vi "VCPAM_CTRL(Host)v2.vi"() -> ()   [LabVIEW 2011]
uses:
  AlazarTech/ATS-VI/5.8.3/ATS_ctl/ATS_DMA_Channel.ctl
  <vilib>/userDefined/High Color/nirio_resource_hc.ctl
  AlazarTech/ATS-VI/5.8.3/ATS_ctl/ATS_Async_Ctrl.ctl
  AlazarTech/ATS-VI/5.8.3/ATS_ctl/Device_Ctrl.ctl
  <vilib>/FPGAPlugInAG/PCI-7830R/niLvFpga_Open_PCI-7830R.vi
  <vilib>/FPGAPlugInAG/PCI-7830R/niLvFpga_Reset_PCI-7830R.vi
  <vilib>/Utility/error.llb/Error Cluster From Error Code.vi
  <vilib>/rvi/errors/niLvFpgaAdjustHostInterfaceError.vi
  <vilib>/FPGAPlugInAG/PCI-7830R/niLvFpga_Run_PCI-7830R.vi
  <vilib>/RVI Host/nirviSupport.llb/nirviErrorClusterFromErrorCode.vi
  <vilib>/Analysis/baseanly.llb/Normalize Vector.vi
  <vilib>/FPGAPlugInAG/PCI-7830R/niLvFpga_Close_PCI-7830R.vi
  <vilib>/rvi/interface/nirviOpenFPGA/nirviOpenFPGA.xnode
  FPGA Bitfiles/VoiceCoilPAMFPGA_FPGATarget_VCPAMCTRL(FPGA)_292315D5.lvbitx
  VCPAM_CTRL(FPGA).vi
  <vilib>/rvi/interface/nirviMethod/nirviMethod.xnode
  <vilib>/rvi/interface/nirviReadWriteControl/nirviReadWriteControl.xnode
  <vilib>/rvi/interface/nirviCloseFPGA/nirviCloseFPGA.xnode
  <vilib>/Analysis/NI_AALPro.lvlib
  <vilib>/Analysis/NI_AALBase.lvlib
  <vilib>/rvi/errors/niLvFpgaMergeErrorWithErrorCode.vi
  <vilib>/FPGAPlugInAG/PCI-7830R/niLvFpga_ConfigureFifo_PCI-7830R.vi
  <vilib>/FPGAPlugInAG/PCI-7830R/niLvFpga_WriteFifo_PCI-7830R.vi
  NiFpgaLv.dll
  <vilib>/FPGAPlugInAG/PCI-7830R/niLvFpga_AcknowledgeIrq_PCI-7830R.vi
  <vilib>/rvi/interface/nirviMethod/StockFPGA_InlinedMethodWaitForMultipleIRQ.vi
  <vilib>/FPGAPlugInAG/PCI-7830R/niLvFpga_WaitOnIrq_PCI-7830R.vi
panel:
  in  "AuxPreTime":u8=15
  in  "CutTail":dbl
  in  "step_delay":u32
  in  "Phase0(deg)":dbl=82.0 format="%0.2f"
  in  "TrigPW":u32
  out "Tri_pt_sent":i32=805864
  in  "Voice Coil PAM Imaging Controller":enum32{"Main", "Tune Voice Coil", "Others"}(tab)
  in  "bscan repeat":i32=1
  in  "Savemap":bool=TRUE
  in  "even step":bool
  in  "load flow":bool
  in  "Save Setting":bool
  in  "Load SO2":bool
  out "MAP":dbl[][](graph)
  in  "MAP Disp":bool=TRUE
  in  "signal type":T1(ring)
  in  "x (mm)":dbl=5.0 format="%0.2f"
  in  "B-scan Rate":dbl=160.0 min=0.1 max=1000.0 step=0.1 format="%#_4g"
  in  "B-scan #":dbl=100.0
  in  "Y Step Size":dbl=16.0
  in  "3D scan #":dbl=300.0
  in  "Ele_Ini_Dir":bool=TRUE caption="Motor"
  in  "Elevational Mode":enum32{"Continuous", "Discrete"}(radio)
  in  "Bi_Dir_Scan":bool=TRUE
  in  "Laser Rep Rate":u32=200000
  in  "Dual Laser":bool
  out "Ele_pt_sent":i32=10978
  out "B-Scan Pos":i32=-936
  in  "Y Enable":bool=TRUE
  in  "Move x":bool
  in  "Move y":bool
  in  "Left":bool
  out "x step motor pos":i32
  in  "Pt per A-line":i32=128
  out "PLL Locked":bool
  in  "Channel":T2
  in  "Trig. Delay (us)":sgl=4.3
  out "DAQ Error":bool
  out "Error source":string="ATS :     ApiSuccess"
  in  "Display Data Per             Frm":bool=TRUE
  in  "file path":path=path "C:/Users/MEMS-PAM/My Data/2013-03-07/2.dat"
  in  "Save Data":bool=TRUE
  in  "acc_PA":bool=TRUE
  out "B-scan saved":i32=684
  out "B-scan displayed":i32=684
  in  "EveryFrm":i32 format="%b"
  in  "Pulse_Out_En":bool
  out "B-Scan":u16[][](graph)
  out "Alines":i32=1176
  in  "start":i32
  in  "depth":i32=128
  out "PD":u16[](graph)
  in  "Ele_StepM_En":bool
  in  "xsteps":i32
  in  "x0 (mm)":dbl format="%0.4f"
  out "x-y":u32=36
  in  "catbscan":i16=6
  in  "stop":bool
  out "data_fetch_finished":bool
  out "stop_disp":bool=TRUE
  in  "showmap":bool=TRUE
  in  "A/B-line show":bool=TRUE
  out "Vocie-coil Traj":i16[](graph)=[6490, 6495, 6499, 6504, 6508, 6512, 6516, 6519, 6523, 6526, 6529, 6532, 6535, 6537, 6540, 6542, 6544, 6546, 6547, 6549, 6550, 6551, 6552, 6553, 6553, 6553, 6554, 6554, 6553, 6553, 6552, 6551, 6550, 6549, 6548, 6546, 6544, 6543, 6540, 6538, 6536, 6533, 6530, 6527, 6524, 6520, 6517, 6513, 6509, 6505, 6500, 6496, 6491, 6486, 6481, 6476, 6470, 6465, 6459, 6453, 6447, 6440, 6434, 6427, 6420, 6413, 6405, 6398, 6390, 6382, 6374, 6366, 6358, 6349, 6340, 6331, 6322, 6313, 6304, 6294, 6284, 6274, 6264, 6253, 6243, 6232, 6221, 6210, 6199, 6187, 6176, 6164, 6152, 6140, 6127, 6115, 6102, 6089, 6076, 6063, 6050, 6036, 6023, 6009, 5995, 5980, 5966, 5951, 5937, 5922, 5907, 5891, 5876, 5860, 5845, 5829, 5813, 5796, 5780, 5763, 5747, 5730, 5713, 5695, 5678, 5660, 5643, 5625, 5607, 5588, 5570, 5552, 5533, 5514, 5495, 5476, 5457, 5437, 5417, 5398, 5378, 5358, 5337, 5317, 5296, 5276, 5255, 5234, 5213, 5191, 5170, 5148, 5127, 5105, 5083, 5061, 5038, 5016, 4993, 4970, 4948, 4925, 4901, 4878, 4855, 4831, 4807, 4783, 4759, 4735, 4711, 4687, 4662, 4637, 4613, 4588, 4563, 4537, 4512, 4487, 4461, 4435, 4409, 4383, 4357, 4331, 4305, 4278, 4252, 4225, 4198, 4171, 4144, 4117, 4090, 4062, 4035, 4007, 3979, 3952, 3924, 3895, 3867, 3839, 3810, 3782, 3753, 3724, 3696, 3667, 3638, 3608, 3579, 3550, 3520, 3491, 3461, 3431, 3401, 3371, 3341, 3311, 3281, 3250, 3220, 3189, 3159, 3128, 3097, 3066, 3035, 3004, 2973, 2942, 2911, 2879, 2848, 2816, 2784, 2753, 2721, 2689, 2657, 2625, 2593, 2561, 2528, 2496, 2464, 2431, 2399, 2366, 2333, 2301, 2268, 2235, 2202, 2169, 2136, 2103, 2070, 2036, 2003, 1970, 1936, 1903, 1869, 1836, 1802, 1768, 1734, 1701, 1667, 1633, 1599, 1565, 1531, 1497, 1463, 1429, 1395, 1360, 1326, 1292, 1257, 1223, 1189, 1154, 1120, 1085, 1051, 1016, 981, 947, 912, 877, 843, 808, 773, 738, 704, 669, 634, 599, 564, 529, 494, 459, 425, 390, 355, 320, 285, 250, 215, 180, 145, 110, 75, 40, 5, -30, -65, -100, -135, -170, -205, -240, -275, -310, -345, -380, -415, -450, -485, -520, -555, -590, -625, -659, -694, -729, -764, -799, -833, -868, -903, -938, -972, -1007, -1041, -1076, -1110, -1145, -1179, -1214, -1248, -1283, -1317, -1351, -1385, -1420, -1454, -1488, -1522, -1556, -1590, -1624, -1658, -1692, -1725, -1759, -1793, -1827, -1860, -1894, -1927, -1961, -1994, -2027, -2061, -2094, -2127, -2160, -2193, -2226, -2259, -2292, -2325, -2357, -2390, -2423, -2455, -2487, -2520, -2552, -2584, -2616, -2649, -2681, -2712, -2744, -2776, -2808, -2839, -2871, -2902, -2934, -2965, -2996, -3027, -3058, -3089, -3120, -3151, -3181, -3212, -3242, -3273, -3303, -3333, -3363, -3393, -3423, -3453, -3483, -3512, -3542, -3571, -3601, -3630, -3659, -3688, -3717, -3746, -3774, -3803, -3831, -3860, -3888, -3916, -3944, -3972, -4000, -4027, -4055, -4082, -4110, -4137, -4164, -4191, -4218, -4245, -4271, -4298, -4324, -4350, -4377, -4403, -4428, -4454, -4480, -4505, -4531, -4556, -4581, -4606, -4631, -4656, -4680, -4705, -4729, -4753, -4777, -4801, -4825, -4848, -4872, -4895, -4918, -4941, -4964, -4987, -5010, -5032, -5055, -5077, -5099, -5121, -5143, -5164, -5186, -5207, -5228, -5249, -5270, -5291, -5312, -5332, -5352, -5372, -5392, -5412, -5432, -5451, -5471, -5490, -5509, -5528, -5547, -5565, -5584, -5602, -5620, -5638, -5656, -5673, -5691, -5708, -5725, -5742, -5759, -5775, -5792, -5808, -5824, -5840, -5856, -5872, -5887, -5903, -5918, -5933, -5947, -5962, -5977, -5991, -6005, -6019, -6033, -6046, -6060, -6073, -6086, -6099, -6112, -6124, -6137, -6149, -6161, -6173, -6184, -6196, -6207, -6218, -6229, -6240, -6251, -6261, -6271, -6281, -6291, -6301, -6311, -6320, -6329, -6338, -6347, -6356, -6364, -6372, -6380, -6388, -6396, -6404, -6411, -6418, -6425, -6432, -6438, -6445, -6451, -6457, -6463, -6469, -6474, -6480, -6485, -6490, -6495, -6499, -6504, -6508, -6512, -6516, -6519, -6523, -6526, -6529, -6532, -6535, -6537, -6540, -6542, -6544, -6546, -6547, -6549, -6550, -6551, -6552, -6553, -6553, -6553, -6554, -6554, -6553, -6553, -6552, -6551, -6550, -6549, -6548, -6546, -6544, -6543, -6540, -6538, -6536, -6533, -6530, -6527, -6524, -6520, -6517, -6513, -6509, -6505, -6500, -6496, -6491, -6486, -6481, -6476, -6470, -6465, -6459, -6453, -6447, -6440, -6434, -6427, -6420, -6413, -6405, -6398, -6390, -6382, -6374, -6366, -6358, -6349, -6340, -6331, -6322, -6313, -6304, -6294, -6284, -6274, -6264, -6253, -6243, -6232, -6221, -6210, -6199, -6187, -6176, -6164, -6152, -6140, -6127, -6115, -6102, -6089, -6076, -6063, -6050, -6036, -6023, -6009, -5995, -5980, -5966, -5951, -5937, -5922, -5907, -5891, -5876, -5860, -5845, -5829, -5813, -5796, -5780, -5763, -5747, -5730, -5713, -5695, -5678, -5660, -5643, -5625, -5607, -5588, -5570, -5552, -5533, -5514, -5495, -5476, -5457, -5437, -5417, -5398, -5378, -5358, -5337, -5317, -5296, -5276, -5255, -5234, -5213, -5191, -5170, -5148, -5127, -5105, -5083, -5061, -5038, -5016, -4993, -4970, -4948, -4925, -4901, -4878, -4855, -4831, -4807, -4783, -4759, -4735, -4711, -4687, -4662, -4637, -4613, -4588, -4563, -4537, -4512, -4487, -4461, -4435, -4409, -4383, -4357, -4331, -4305, -4278, -4252, -4225, -4198, -4171, -4144, -4117, -4090, -4062, -4035, -4007, -3979, -3952, -3924, -3895, -3867, -3839, -3810, -3782, -3753, -3724, -3696, -3667, -3638, -3608, -3579, -3550, -3520, -3491, -3461, -3431, -3401, -3371, -3341, -3311, -3281, -3250, -3220, -3189, -3159, -3128, -3097, -3066, -3035, -3004, -2973, -2942, -2911, -2879, -2848, -2816, -2784, -2753, -2721, -2689, -2657, -2625, -2593, -2561, -2528, -2496, -2464, -2431, -2399, -2366, -2333, -2301, -2268, -2235, -2202, -2169, -2136, -2103, -2070, -2036, -2003, -1970, -1936, -1903, -1869, -1836, -1802, -1768, -1734, -1701, -1667, -1633, -1599, -1565, -1531, -1497, -1463, -1429, -1395, -1360, -1326, -1292, -1257, -1223, -1189, -1154, -1120, -1085, -1051, -1016, -981, -947, -912, -877, -843, -808, -773, -738, -704, -669, -634, -599, -564, -529, -494, -459, -425, -390, -355, -320, -285, -250, -215, -180, -145, -110, -75, -40, -5, 30, 65, 100, 135, 170, 205, 240, 275, 310, 345, 380, 415, 450, 485, 520, 555, 590, 625, 659, 694, 729, 764, 799, 833, 868, 903, 938, 972, 1007, 1041, 1076, 1110, 1145, 1179, 1214, 1248, 1283, 1317, 1351, 1385, 1420, 1454, 1488, 1522, 1556, 1590, 1624, 1658, 1692, 1725, 1759, 1793, 1827, 1860, 1894, 1927, 1961, 1994, 2027, 2061, 2094, 2127, 2160, 2193, 2226, 2259, 2292, 2325, 2357, 2390, 2423, 2455, 2487, 2520, 2552, 2584, 2616, 2649, 2681, 2712, 2744, 2776, 2808, 2839, 2871, 2902, 2934, 2965, 2996, 3027, 3058, 3089, 3120, 3151, 3181, 3212, 3242, 3273, 3303, 3333, 3363, 3393, 3423, 3453, 3483, 3512, 3542, 3571, 3601, 3630, 3659, 3688, 3717, 3746, 3774, 3803, 3831, 3860, 3888, 3916, 3944, 3972, 4000, 4027, 4055, 4082, 4110, 4137, 4164, 4191, 4218, 4245, 4271, 4298, 4324, 4350, 4377, 4403, 4428, 4454, 4480, 4505, 4531, 4556, 4581, 4606, 4631, 4656, 4680, 4705, 4729, 4753, 4777, 4801, 4825, 4848, 4872, 4895, 4918, 4941, 4964, 4987, 5010, 5032, 5055, 5077, 5099, 5121, 5143, 5164, 5186, 5207, 5228, 5249, 5270, 5291, 5312, 5332, 5352, 5372, 5392, 5412, 5432, 5451, 5471, 5490, 5509, 5528, 5547, 5565, 5584, 5602, 5620, 5638, 5656, 5673, 5691, 5708, 5725, 5742, 5759, 5775, 5792, 5808, 5824, 5840, 5856, 5872, 5887, 5903, 5918, 5933, 5947, 5962, 5977, 5991, 6005, 6019, 6033, 6046, 6060, 6073, 6086, 6099, 6112, 6124, 6137, 6149, 6161, 6173, 6184, 6196, 6207, 6218, 6229, 6240, 6251, 6261, 6271, 6281, 6291, 6301, 6311, 6320, 6329, 6338, 6347, 6356, 6364, 6372, 6380, 6388, 6396, 6404, 6411, 6418, 6425, 6432, 6438, 6445, 6451, 6457, 6463, 6469, 6474, 6480, 6485]
  out "VC_POS":i16[](graph)
  in  "AcqVCPos":bool
  in  "Calc_delay":bool
  out "VC_In":dbl[](graph)=[1.0, 0.9999857270394815, 0.999942908565361, 0.9998715457999312, 0.999771640780308, 0.9996431963583721, 0.9994862162006879, 0.9993007047883986, 0.9990866674170983, 0.9988441101966808, 0.9985730400511657, 0.9982734647184995, 0.9979453927503363, 0.9975888335117926, 0.9972037971811801, 0.9967902947497157, 0.9963483380212069, 0.9958779396117159, 0.9953791129491981, 0.9948518722731206, 0.9942962326340535, 0.9937122098932426, 0.9930998207221545, 0.9924590826020026, 0.991790013823246, 0.99109263348507, 0.990366961494838, 0.9896130185675259, 0.9888308262251285, 0.988020406796047, 0.9871817834144501, 0.9863149800196149, 0.9854200213552425, 0.9844969329687524, 0.9835457412105527, 0.9825664732332882, 0.9815591569910653, 0.9805238212386539, 0.9794604955306667, 0.9783692102207152, 0.977249996460544, 0.9761028861991403, 0.9749279121818236, 0.9737251079493088, 0.9724945078367512, 0.9712361469727636, 0.9699500612784169, 0.9686362874662107, 0.9672948630390295, 0.9659258262890681, 0.9645292162967425, 0.9631050729295701, 0.9616534368410363, 0.960174349469429, 0.9586678530366607, 0.9571339905470584, 0.9555728057861408, 0.9539843433193637, 0.9523686484908522, 0.9507257674221025, 0.9490557470106686, 0.9473586349288206, 0.9456344796221867, 0.9438833303083672, 0.9421052369755334, 0.9403002503809957, 0.9384684220497604, 0.936609804273053, 0.9347244501068311, 0.9328124133702644, 0.9308737486442044, 0.9289085112696193, 0.9269167573460219, 0.9248985437298606, 0.9228539280329038, 0.9207829686205878, 0.9186857246103585, 0.9165622558699758, 0.9144126230158125, 0.9122368874111166, 0.9100351111642666, 0.9078073571269917, 0.9055536888925844, 0.9032741707940783, 0.9009688679024191, 0.8986378460245992, 0.8962811717017867, 0.8938989122074191, 0.8914911355452896, 0.8890579104475989, 0.8865993063730001, 0.8841153935046094, 0.8816062427480091, 0.8790719257292169, 0.8765125147926478, 0.8739280829990428, 0.8713187041233894, 0.8686844526528094, 0.8660254037844387, 0.8633416334232749, 0.8606332181800164, 0.8579002353688691, 0.8551427630053463, 0.8523608798040346, 0.849554665176354, 0.8467241992282839, 0.8438695627580834, 0.8409908372539782, 0.8380881048918408, 0.8351614485328384, 0.832210951721074, 0.8292366986811948, 0.826238774315995, 0.8232172642039852, 0.820172254596956, 0.8171038324175097, 0.814012085256585, 0.8108971013709507, 0.8077589696806924, 0.8045977797666681, 0.8014136218679567, 0.798206586879277, 0.7949767663483978, 0.7917242524735195, 0.7884491381006479, 0.7851515167209376, 0.7818314824680299, 0.7784891301153587, 0.7751245550734519, 0.7717378533872015, 0.7683291217331278, 0.7648984574166141, 0.7614459583691345, 0.7579717231454527, 0.7544758509208145, 0.750958441488111, 0.7474195952550354, 0.7438594132412116, 0.7402779970753156, 0.736675448992169, 0.7330518718298265, 0.7294073690266338, 0.7257420446182822, 0.7220560032348308, 0.7183493500977277, 0.714622191016799, 0.7108746323872351, 0.7071067811865472, 0.7033187449715197, 0.6995106318751337, 0.6956825506034865, 0.6918346104326822, 0.6879669212057188, 0.6840795933293458, 0.6801727377709195, 0.6762464660552285, 0.6723008902613169, 0.668336123019278, 0.6643522775070462, 0.660349467447159, 0.6563278071035183, 0.6522874112781208, 0.6482283953077885, 0.644150875060869, 0.640054966933935, 0.6359407878484549, 0.6318084552474614, 0.6276580870921933, 0.6234898018587336, 0.6193037185346221, 0.615099956615464, 0.610878636101514, 0.6066398774942554, 0.6023838017929554, 0.5981105304912161, 0.5938201855735014, 0.5895128895116599, 0.5851887652614235, 0.580847936258903, 0.5764905264170588, 0.5721166601221698, 0.5677264622302762, 0.5633200580636222, 0.5588975734070712, 0.554459134504523, 0.5500048680553021, 0.5455349012105488, 0.5410493615695817, 0.5365483771762631, 0.5320320765153362, 0.527500588508765, 0.5229540425120464, 0.5183925683105252, 0.5138162961156819, 0.5092253565614233, 0.5046198807003452, 0.5000000000000002, 0.49536584633913555, 0.49071755200393813, 0.48605524968424857, 0.4813790724697832, 0.47668915384632504, 0.47198562769192326, 0.46726862827306165, 0.46253829024083554, 0.45779474862709846, 0.4530381388406172, 0.4482685966631967, 0.4434862582458137, 0.4386912601047207, 0.4338837391175584, 0.4290638325194388, 0.4242316778990376, 0.41938741319465644, 0.41453117669029566, 0.4096631070116965, 0.40478334312239406, 0.39989202431974064, 0.39498929023093887, 0.3900752808090466, 0.38515013632899103, 0.3802139973835553, 0.37526700487937437, 0.3703093000329032, 0.36534102436639526, 0.360362319703853, 0.355373328166989, 0.3503741921711594, 0.3453650544213078, 0.34034605790788275, 0.3353173459027645, 0.33027906195516676, 0.32523134988754737, 0.3201743537914943, 0.31510821802362093, 0.3100330872014367, 0.3049491061992275, 0.29985642014391134, 0.2947551744109045, 0.2896455146199625, 0.2845275866310327, 0.27940153654008093, 0.2742675106749307, 0.26912565559107654, 0.2639761180675101, 0.25881904510252046, 0.2536545839095077, 0.2484828819127708, 0.24330408674330897, 0.23811834623459788, 0.23292580841837887, 0.22772662152042417, 0.22252093395631467, 0.2173088943271943, 0.21209065141553693, 0.20686635418089053, 0.20163615175563354, 0.19640019344070933, 0.19115862870137254, 0.18591160716291433, 0.1806592786063992, 0.17540179296438138, 0.17013930031663288, 0.16487195088585127, 0.15959989503337946, 0.15432328325490557, 0.1490422661761747, 0.14375699454868143, 0.13846761924537423, 0.13317429125634095, 0.12787716168450625, 0.12257638174131076, 0.117272102742402, 0.11196447610330765, 0.10665365333512039, 0.10133978604016586, 0.096023025907682, 0.09070352470948198, 0.08538143429562871, 0.08005690659009315, 0.07473009358642448, 0.06940114734340436, 0.06407021998071315, 0.058737463674580714, 0.053403030653449146, 0.048067073193620594, 0.042729743614917, 0.03739119427632544, 0.03205157757165539, 0.02671104592518208, 0.02136975178730176, 0.01602784763017357, 0.010685485943373305, 0.005342819229534299, 2.0499976092743302e-16, -0.005342819229534634, -0.010685485943372895, -0.016027847630173904, -0.021369751787301352, -0.026711045925182413, -0.03205157757165498, -0.03739119427632577, -0.04272974361491659, -0.04806707319362093, -0.05340303065344874, -0.05873746367458105, -0.06407021998071273, -0.06940114734340469, -0.07473009358642406, -0.08005690659009349, -0.08538143429562829, -0.09070352470948231, -0.09602302590768158, -0.10133978604016619, -0.10665365333511997, -0.11196447610330798, -0.1172721027424016, -0.1225763817413111, -0.12787716168450583, -0.13317429125634128, -0.13846761924537382, -0.14375699454868177, -0.14904226617617428, -0.1543232832549059, -0.15959989503337907, -0.1648719508858516, -0.1701393003166325, -0.17540179296438171, -0.1806592786063988, -0.18591160716291466, -0.19115862870137215, -0.19640019344070966, -0.20163615175563315, -0.20686635418089086, -0.21209065141553654, -0.21730889432719463, -0.22252093395631428, -0.2277266215204245, -0.23292580841837848, -0.2381183462345982, -0.24330408674330858, -0.24848288191277113, -0.2536545839095073, -0.2588190451025208, -0.2639761180675097, -0.2691256555910769, -0.2742675106749303, -0.27940153654008126, -0.28452758663103234, -0.28964551461996285, -0.2947551744109041, -0.2998564201439117, -0.3049491061992271, -0.310033087201437, -0.31510821802362055, -0.3201743537914946, -0.325231349887547, -0.3302790619551671, -0.33531734590276413, -0.3403460579078831, -0.34536505442130744, -0.3503741921711597, -0.35537332816698863, -0.36036231970385335, -0.3653410243663949, -0.3703093000329035, -0.375267004879374, -0.38021399738355566, -0.38515013632899064, -0.3900752808090469, -0.3949892902309385, -0.39989202431974097, -0.40478334312239367, -0.40966310701169684, -0.41453117669029527, -0.4193874131946568, -0.4242316778990372, -0.42906383251943914, -0.433883739117558, -0.43869126010472104, -0.44348625824581334, -0.448268596663197, -0.45303813884061683, -0.4577947486270988, -0.46253829024083515, -0.467268628273062, -0.47198562769192287, -0.4766891538463254, -0.4813790724697828, -0.4860552496842489, -0.49071755200393774, -0.4953658463391359, -0.49999999999999983, -0.5046198807003456, -0.509225356561423, -0.5138162961156822, -0.5183925683105248, -0.5229540425120467, -0.5275005885087647, -0.5320320765153366, -0.5365483771762628, -0.541049361569582, -0.5455349012105485, -0.5500048680553025, -0.5544591345045227, -0.5588975734070716, -0.5633200580636218, -0.5677264622302766, -0.5721166601221694, -0.5764905264170591, -0.5808479362589026, -0.5851887652614238, -0.5895128895116596, -0.5938201855735017, -0.5981105304912158, -0.6023838017929557, -0.6066398774942551, -0.6108786361015144, -0.6150999566154637, -0.6193037185346224, -0.6234898018587333, -0.6276580870921936, -0.6318084552474611, -0.6359407878484552, -0.6400549669339347, -0.6441508750608693, -0.6482283953077882, -0.6522874112781212, -0.656327807103518, -0.6603494674471594, -0.6643522775070458, -0.6683361230192784, -0.6723008902613166, -0.6762464660552289, -0.6801727377709191, -0.6840795933293461, -0.6879669212057185, -0.6918346104326826, -0.6956825506034862, -0.6995106318751341, -0.7033187449715194, -0.7071067811865476, -0.7108746323872348, -0.7146221910167994, -0.7183493500977274, -0.7220560032348311, -0.7257420446182818, -0.7294073690266342, -0.7330518718298261, -0.7366754489921693, -0.7402779970753154, -0.743859413241212, -0.7474195952550352, -0.7509584414881113, -0.7544758509208143, -0.757971723145453, -0.7614459583691343, -0.7648984574166144, -0.7683291217331276, -0.7717378533872018, -0.7751245550734517, -0.778489130115359, -0.7818314824680297, -0.785151516720938, -0.7884491381006477, -0.7917242524735199, -0.7949767663483975, -0.7982065868792774, -0.8014136218679565, -0.8045977797666685, -0.8077589696806922, -0.8108971013709511, -0.8140120852565847, -0.8171038324175101, -0.8201722545969558, -0.8232172642039856, -0.8262387743159948, -0.8292366986811951, -0.8322109517210737, -0.8351614485328387, -0.8380881048918406, -0.8409908372539785, -0.8438695627580832, -0.8467241992282842, -0.8495546651763538, -0.852360879804035, -0.8551427630053461, -0.8579002353688694, -0.8606332181800161, -0.8633416334232752, -0.8660254037844386, -0.8686844526528097, -0.8713187041233893, -0.8739280829990431, -0.8765125147926477, -0.8790719257292171, -0.881606242748009, -0.8841153935046097, -0.886599306373, -0.8890579104475991, -0.8914911355452895, -0.8938989122074193, -0.8962811717017866, -0.8986378460245994, -0.900968867902419, -0.9032741707940786, -0.9055536888925843, -0.9078073571269919, -0.9100351111642665, -0.9122368874111169, -0.9144126230158124, -0.916562255869976, -0.9186857246103584, -0.9207829686205881, -0.9228539280329037, -0.9248985437298608, -0.9269167573460217, -0.9289085112696195, -0.9308737486442042, -0.9328124133702647, -0.934724450106831, -0.9366098042730532, -0.9384684220497604, -0.940300250380996, -0.9421052369755334, -0.9438833303083675, -0.9456344796221867, -0.9473586349288208, -0.9490557470106686, -0.9507257674221027, -0.9523686484908522, -0.9539843433193639, -0.9555728057861408, -0.9571339905470586, -0.9586678530366607, -0.9601743494694293, -0.9616534368410363, -0.9631050729295704, -0.9645292162967425, -0.9659258262890683, -0.9672948630390295, -0.9686362874662109, -0.9699500612784169, -0.9712361469727638, -0.9724945078367512, -0.973725107949309, -0.9749279121818236, -0.9761028861991405, -0.977249996460544, -0.9783692102207153, -0.9794604955306667, -0.980523821238654, -0.9815591569910653, -0.9825664732332883, -0.9835457412105527, -0.9844969329687524, -0.9854200213552425, -0.9863149800196149, -0.9871817834144502, -0.988020406796047, -0.9888308262251286, -0.9896130185675259, -0.9903669614948382, -0.99109263348507, -0.9917900138232462, -0.9924590826020026, -0.9930998207221546, -0.9937122098932426, -0.9942962326340536, -0.9948518722731206, -0.9953791129491982, -0.9958779396117159, -0.996348338021207, -0.9967902947497157, -0.9972037971811802, -0.9975888335117926, -0.9979453927503364, -0.9982734647184995, -0.9985730400511658, -0.9988441101966808, -0.9990866674170984, -0.9993007047883985, -0.999486216200688, -0.999643196358372, -0.9997716407803081, -0.9998715457999311, -0.9999429085653612, -0.9999857270394814, -1.0, -0.9999857270394814, -0.999942908565361, -0.9998715457999311, -0.999771640780308, -0.999643196358372, -0.9994862162006879, -0.9993007047883984, -0.9990866674170983, -0.9988441101966806, -0.9985730400511657, -0.9982734647184993, -0.9979453927503363, -0.9975888335117924, -0.9972037971811801, -0.9967902947497155, -0.9963483380212069, -0.9958779396117157, -0.9953791129491982, -0.9948518722731203, -0.9942962326340536, -0.9937122098932424, -0.9930998207221546, -0.9924590826020023, -0.9917900138232462, -0.9910926334850698, -0.9903669614948382, -0.9896130185675257, -0.9888308262251286, -0.9880204067960467, -0.9871817834144502, -0.9863149800196147, -0.9854200213552426, -0.9844969329687522, -0.9835457412105528, -0.9825664732332879, -0.9815591569910654, -0.9805238212386537, -0.9794604955306668, -0.978369210220715, -0.9772499964605441, -0.9761028861991401, -0.9749279121818237, -0.9737251079493086, -0.9724945078367513, -0.9712361469727634, -0.969950061278417, -0.9686362874662104, -0.9672948630390296, -0.9659258262890679, -0.9645292162967426, -0.9631050729295699, -0.9616534368410364, -0.9601743494694288, -0.9586678530366608, -0.9571339905470582, -0.9555728057861409, -0.9539843433193634, -0.9523686484908523, -0.9507257674221022, -0.9490557470106687, -0.9473586349288203, -0.9456344796221868, -0.943883330308367, -0.9421052369755335, -0.9403002503809955, -0.9384684220497606, -0.9366098042730527, -0.9347244501068313, -0.9328124133702642, -0.9308737486442045, -0.928908511269619, -0.926916757346022, -0.9248985437298604, -0.9228539280329039, -0.9207829686205876, -0.9186857246103586, -0.9165622558699755, -0.9144126230158126, -0.9122368874111164, -0.9100351111642667, -0.9078073571269915, -0.9055536888925845, -0.9032741707940781, -0.9009688679024193, -0.898637846024599, -0.8962811717017868, -0.8938989122074189, -0.8914911355452897, -0.8890579104475986, -0.8865993063730002, -0.8841153935046092, -0.8816062427480093, -0.8790719257292166, -0.8765125147926479, -0.8739280829990425, -0.8713187041233895, -0.868684452652809, -0.8660254037844388, -0.8633416334232745, -0.8606332181800165, -0.8579002353688687, -0.8551427630053464, -0.8523608798040343, -0.8495546651763541, -0.8467241992282836, -0.8438695627580836, -0.8409908372539778, -0.8380881048918409, -0.835161448532838, -0.8322109517210741, -0.8292366986811944, -0.8262387743159951, -0.8232172642039849, -0.8201722545969561, -0.8171038324175094, -0.8140120852565851, -0.8108971013709504, -0.8077589696806926, -0.8045977797666677, -0.801413621867957, -0.7982065868792766, -0.794976766348398, -0.7917242524735191, -0.7884491381006481, -0.7851515167209372, -0.7818314824680301, -0.7784891301153583, -0.7751245550734521, -0.771737853387201, -0.7683291217331281, -0.7648984574166137, -0.7614459583691348, -0.7579717231454522, -0.7544758509208147, -0.7509584414881105, -0.7474195952550357, -0.7438594132412112, -0.7402779970753158, -0.7366754489921685, -0.7330518718298267, -0.7294073690266334, -0.7257420446182824, -0.7220560032348303, -0.7183493500977279, -0.7146221910167986, -0.7108746323872354, -0.7071067811865468, -0.7033187449715199, -0.6995106318751333, -0.6956825506034867, -0.6918346104326818, -0.687966921205719, -0.6840795933293453, -0.6801727377709197, -0.6762464660552281, -0.6723008902613171, -0.6683361230192776, -0.6643522775070464, -0.6603494674471586, -0.6563278071035186, -0.6522874112781204, -0.6482283953077888, -0.6441508750608685, -0.6400549669339353, -0.6359407878484544, -0.6318084552474617, -0.6276580870921928, -0.6234898018587338, -0.6193037185346216, -0.6150999566154642, -0.6108786361015136, -0.6066398774942556, -0.6023838017929549, -0.5981105304912163, -0.5938201855735009, -0.5895128895116601, -0.585188765261423, -0.5808479362589032, -0.5764905264170583, -0.57211666012217, -0.5677264622302758, -0.5633200580636224, -0.5588975734070708, -0.5544591345045232, -0.5500048680553017, -0.545534901210549, -0.5410493615695813, -0.5365483771762634, -0.5320320765153358, -0.5275005885087652, -0.5229540425120459, -0.5183925683105254, -0.5138162961156815, -0.5092253565614235, -0.5046198807003448, -0.5000000000000004, -0.4953658463391351, -0.49071755200393835, -0.4860552496842481, -0.4813790724697834, -0.4766891538463246, -0.4719856276919235, -0.4672686282730612, -0.46253829024083576, -0.457794748627098, -0.45303813884061744, -0.44826859666319624, -0.44348625824581395, -0.43869126010472026, -0.4338837391175586, -0.42906383251943836, -0.4242316778990378, -0.419387413194656, -0.4145311766902959, -0.40966310701169606, -0.4047833431223943, -0.3998920243197402, -0.3949892902309391, -0.39007528080904613, -0.38515013632899125, -0.3802139973835549, -0.3752670048793746, -0.37030930003290274, -0.3653410243663955, -0.3603623197038526, -0.35537332816698924, -0.35037419217115895, -0.34536505442130805, -0.3403460579078823, -0.33531734590276474, -0.33027906195516626, -0.3252313498875476, -0.3201743537914938, -0.31510821802362116, -0.3100330872014362, -0.3049491061992277, -0.29985642014391084, -0.2947551744109047, -0.289645514619962, -0.28452758663103295, -0.27940153654008043, -0.27426751067493094, -0.26912565559107604, -0.2639761180675103, -0.25881904510251996, -0.2536545839095079, -0.2484828819127703, -0.2433040867433092, -0.23811834623459738, -0.2329258084183791, -0.22772662152042367, -0.2225209339563149, -0.2173088943271938, -0.21209065141553718, -0.20686635418089003, -0.2016361517556338, -0.19640019344070883, -0.1911586287013728, -0.18591160716291383, -0.18065927860639944, -0.17540179296438088, -0.17013930031663313, -0.16487195088585077, -0.1595998950333797, -0.15432328325490507, -0.14904226617617494, -0.14375699454868093, -0.13846761924537448, -0.13317429125634045, -0.1278771616845065, -0.12257638174131026, -0.11727210274240227, -0.11196447610330715, -0.10665365333512065, -0.10133978604016536, -0.09602302590768226, -0.09070352470948148, -0.08538143429562897, -0.08005690659009265, -0.07473009358642474, -0.06940114734340386, -0.06407021998071341, -0.058737463674580215, -0.05340303065344941, -0.048067073193620094, -0.042729743614917264, -0.03739119427632494, -0.03205157757165566, -0.02671104592518158, -0.021369751787302035, -0.01602784763017307, -0.01068548594337358, -0.0053428192295338, -4.815051962291268e-16, 0.005342819229535133, 0.010685485943372618, 0.016027847630174404, 0.021369751787301074, 0.026711045925182912, 0.0320515775716547, 0.03739119427632627, 0.042729743614916306, 0.048067073193621426, 0.05340303065344845, 0.05873746367458154, 0.06407021998071245, 0.06940114734340519, 0.07473009358642378, 0.08005690659009398, 0.08538143429562801, 0.0907035247094828, 0.0960230259076813, 0.10133978604016668, 0.1066536533351197, 0.11196447610330847, 0.11727210274240131, 0.12257638174131158, 0.12787716168450555, 0.13317429125634175, 0.13846761924537354, 0.14375699454868224, 0.149042266176174, 0.15432328325490638, 0.15959989503337876, 0.16487195088585208, 0.17013930031663219, 0.17540179296438219, 0.1806592786063985, 0.18591160716291513, 0.19115862870137185, 0.19640019344071014, 0.20163615175563285, 0.20686635418089133, 0.21209065141553624, 0.2173088943271951, 0.22252093395631398, 0.22772662152042497, 0.23292580841837818, 0.23811834623459868, 0.24330408674330828, 0.2484828819127716, 0.25365458390950696, 0.25881904510252124, 0.26397611806750937, 0.2691256555910773, 0.27426751067493, 0.2794015365400817, 0.284527586631032, 0.2896455146199633, 0.29475517441090376, 0.29985642014391206, 0.30494910619922677, 0.3100330872014374, 0.3151082180236202, 0.320174353791495, 0.32523134988754665, 0.3302790619551675, 0.3353173459027638, 0.34034605790788347, 0.3453650544213071, 0.3503741921711601, 0.3553733281669883, 0.36036231970385374, 0.36534102436639454, 0.3703093000329039, 0.37526700487937364, 0.38021399738355605, 0.3851501363289903, 0.3900752808090473, 0.39498929023093815, 0.39989202431974136, 0.40478334312239334, 0.4096631070116972, 0.41453117669029493, 0.41938741319465717, 0.4242316778990369, 0.4290638325194395, 0.4338837391175577, 0.4386912601047214, 0.443486258245813, 0.4482685966631974, 0.4530381388406165, 0.4577947486270992, 0.4625382902408348, 0.46726862827306237, 0.47198562769192254, 0.47668915384632576, 0.48137907246978245, 0.4860552496842493, 0.4907175520039374, 0.4953658463391363, 0.4999999999999995, 0.504619880700346, 0.5092253565614226, 0.5138162961156827, 0.5183925683105245, 0.5229540425120471, 0.5275005885087644, 0.532032076515337, 0.5365483771762625, 0.5410493615695825, 0.5455349012105482, 0.5500048680553029, 0.5544591345045223, 0.558897573407072, 0.5633200580636215, 0.567726462230277, 0.5721166601221691, 0.5764905264170596, 0.5808479362589023, 0.5851887652614242, 0.5895128895116593, 0.593820185573502, 0.5981105304912154, 0.602383801792956, 0.6066398774942547, 0.6108786361015147, 0.6150999566154634, 0.6193037185346227, 0.6234898018587329, 0.627658087092194, 0.6318084552474608, 0.6359407878484555, 0.6400549669339344, 0.6441508750608697, 0.6482283953077879, 0.6522874112781215, 0.6563278071035177, 0.6603494674471597, 0.6643522775070455, 0.6683361230192787, 0.6723008902613162, 0.6762464660552292, 0.6801727377709188, 0.6840795933293464, 0.6879669212057181, 0.6918346104326829, 0.6956825506034858, 0.6995106318751344, 0.703318744971519, 0.7071067811865479, 0.7108746323872345, 0.7146221910167997, 0.718349350097727, 0.7220560032348314, 0.7257420446182815, 0.7294073690266345, 0.7330518718298258, 0.7366754489921696, 0.740277997075315, 0.7438594132412122, 0.7474195952550349, 0.7509584414881115, 0.7544758509208139, 0.7579717231454532, 0.761445958369134, 0.7648984574166147, 0.7683291217331273, 0.771737853387202, 0.7751245550734513, 0.7784891301153593, 0.7818314824680294, 0.7851515167209382, 0.7884491381006473, 0.7917242524735201, 0.7949767663483972, 0.7982065868792776, 0.8014136218679562, 0.8045977797666687, 0.8077589696806918, 0.8108971013709513, 0.8140120852565844, 0.8171038324175103, 0.8201722545969554, 0.8232172642039858, 0.8262387743159945, 0.8292366986811953, 0.8322109517210734, 0.8351614485328389, 0.8380881048918403, 0.8409908372539787, 0.8438695627580829, 0.8467241992282845, 0.8495546651763535, 0.8523608798040352, 0.8551427630053458, 0.8579002353688696, 0.8606332181800158, 0.8633416334232754, 0.8660254037844383, 0.8686844526528099, 0.871318704123389, 0.8739280829990433, 0.8765125147926474, 0.8790719257292173, 0.8816062427480087, 0.8841153935046099, 0.8865993063729998, 0.8890579104475993, 0.8914911355452894, 0.8938989122074196, 0.8962811717017864, 0.8986378460245996, 0.9009688679024189, 0.9032741707940788, 0.9055536888925841, 0.9078073571269921, 0.9100351111642664, 0.9122368874111171, 0.9144126230158123, 0.9165622558699762, 0.9186857246103582, 0.9207829686205883, 0.9228539280329036, 0.924898543729861, 0.9269167573460216, 0.9289085112696197, 0.9308737486442041, 0.9328124133702649, 0.9347244501068309, 0.9366098042730534, 0.9384684220497603, 0.9403002503809962, 0.9421052369755333, 0.9438833303083677, 0.9456344796221866, 0.947358634928821, 0.9490557470106685, 0.9507257674221029, 0.9523686484908521, 0.9539843433193641, 0.9555728057861407, 0.9571339905470588, 0.9586678530366606, 0.9601743494694295, 0.9616534368410362, 0.9631050729295706, 0.9645292162967424, 0.9659258262890685, 0.9672948630390293, 0.9686362874662111, 0.9699500612784168, 0.9712361469727641, 0.9724945078367511, 0.9737251079493092, 0.9749279121818235, 0.9761028861991408, 0.9772499964605439, 0.9783692102207155, 0.9794604955306666, 0.9805238212386542, 0.9815591569910652, 0.9825664732332885, 0.9835457412105526, 0.9844969329687526, 0.9854200213552424, 0.9863149800196152, 0.9871817834144501, 0.9880204067960472, 0.9888308262251285, 0.9896130185675261, 0.990366961494838, 0.9910926334850703, 0.991790013823246, 0.9924590826020028, 0.9930998207221545, 0.9937122098932428, 0.9942962326340535, 0.9948518722731208, 0.9953791129491981, 0.9958779396117161, 0.9963483380212069, 0.9967902947497159, 0.9972037971811801, 0.9975888335117928, 0.9979453927503363, 0.9982734647184998, 0.9985730400511657, 0.9988441101966811, 0.9990866674170983, 0.9993007047883987, 0.9994862162006879, 0.9996431963583722, 0.999771640780308, 0.9998715457999313, 0.999942908565361, 0.9999857270394816]
  out "Phase Shift":dbl=-121.17565497157202
  in  "DwnSmpl VCPos":i32=1
  out "VC range":i16=259
  in  "Manual y speed factor":dbl=20.0
  out "Bscan_Steps":u32[](graph)=[212, 205, 198, 189, 180, 170, 161, 151, 142, 133, 124, 116, 109, 101, 96, 91, 88, 84, 82, 79, 77, 76, 75, 74, 73, 72, 72, 72, 72, 72, 72, 72, 72, 72, 72, 72, 72, 72, 72, 72, 72, 72, 72, 72, 72, 72, 72, 72, 72, 72, 72, 72, 72, 72, 72, 72, 72, 72, 72, 72, 72, 72, 72, 72, 72, 72, 72, 72, 72, 72, 72, 72, 72, 72, 72, 72, 72, 72, 72, 72, 72, 72, 72, 72, 72, 72, 72, 72, 72, 72, 72, 72, 72, 72, 72, 72, 72, 72, 72, 72, 72, 72, 72, 72, 72, 72, 72, 72, 72, 72, 72, 72, 72, 72, 72, 72, 72, 72, 72, 72, 72, 72, 72, 72, 72, 72, 72, 72, 72, 72, 72, 72, 72, 72, 72, 72, 72, 72, 72, 72, 72, 72, 72, 72, 72, 72, 72, 72, 72, 72, 72, 72, 72, 72, 72, 72, 72, 72, 72, 72, 72, 72, 72, 72, 72, 72, 72, 72, 72, 72, 72, 72, 72, 72, 72, 72, 72, 72, 72, 72, 72, 72, 72, 72, 72, 72, 72, 72, 72, 72, 72, 72, 72, 72, 72, 72, 72, 72, 72, 72, 72, 72, 72, 72, 72, 72, 72, 72, 72, 72, 72, 72, 72, 72, 72, 72, 72, 72, 72, 72, 72, 72, 72, 72, 72, 72, 72, 72, 72, 72, 72, 72, 72, 72, 72, 72, 72, 72, 72, 72, 72, 72, 72, 72, 72, 72, 72, 72, 72, 72, 72, 72, 72, 72, 72, 72, 72, 72, 72, 72, 72, 72, 72, 72, 72, 72, 72, 72, 72, 72, 72, 72, 72, 72, 72, 72, 72, 72, 72, 72, 72, 72, 72, 72, 72, 72, 72, 72, 72, 72, 72, 72, 72, 72, 72, 72, 72, 72, 72, 72, 72, 72, 72, 72, 72, 72, 72, 72, 72, 72, 72, 72, 72, 72, 72, 72, 72, 72, 72, 72, 72, 72, 72, 72, 72, 72, 72, 72, 72, 72, 72, 72, 72, 72, 72, 72, 72, 72, 72, 72, 72, 72, 72, 72, 72, 72, 72, 72, 72, 72, 72, 72, 72, 72, 72, 72, 72, 72, 72, 72, 72, 72, 72, 72, 72, 72, 72, 72, 72, 72, 72, 72, 72, 72, 72, 72, 72, 72, 72, 72, 72, 72, 72, 72, 72, 72, 72, 72, 72, 72, 72, 72, 72, 72, 72, 72, 72, 72, 72, 72, 72, 72, 72, 72, 72, 72, 72, 72, 72, 72, 72, 72, 72, 72, 72, 72, 72, 72, 72, 72, 72, 72, 72, 72, 72, 72, 72, 72, 72, 72, 72, 72, 72, 72, 72, 72, 72, 72, 72, 72, 72, 72, 72, 72, 72, 72, 72, 72, 72, 72, 72, 72, 72, 72, 72, 72, 72, 72, 72, 72, 72, 72, 72, 72, 72, 72, 72, 72, 72, 72, 72, 72, 72, 72, 72, 72, 72, 72, 72, 72, 72, 72, 72, 72, 72, 72, 72, 72, 72, 72, 72, 72, 72, 72, 72, 72, 72, 72, 72, 72, 72, 72, 72, 72, 72, 72, 72, 72, 72, 72, 72, 72, 72, 72, 72, 72, 72, 72, 72, 72, 72, 72, 72, 72, 72, 72, 72, 72, 72, 72, 72, 72, 72, 72, 72, 72, 72, 72, 72, 72, 72, 72, 72, 72, 72, 72, 72, 72, 72, 72, 72, 72, 72, 72, 72, 72, 72, 72, 72, 72, 72, 72, 72, 72, 72, 72, 72, 72, 72, 72, 72, 72, 72, 72, 72, 72, 72, 72, 72, 72, 72, 72, 72, 72, 72, 72, 72, 72, 72, 72, 72, 72, 72, 72, 72, 72, 72, 72, 72, 72, 72, 72, 72, 72, 72, 72, 72, 72, 72, 72, 72, 72, 72, 72, 72, 72, 72, 72, 72, 72, 72, 72, 72, 72, 72, 72, 72, 72, 72, 72, 72, 72, 72, 72, 72, 72, 72, 72, 72, 72, 72, 72, 72, 72, 72, 72, 72, 72, 72, 72, 72, 72, 72, 72, 72, 72, 72, 72, 72, 72, 72, 72, 72, 72, 72, 72, 72, 72, 72, 72, 72, 72, 72, 72, 72, 72, 72, 72, 72, 72, 72, 72, 72, 72, 72, 72, 72, 72, 72, 72, 72, 72, 72, 72, 72, 72, 72, 72, 72, 72, 72, 72, 72, 72, 72, 72, 72, 72, 72, 72, 72, 72, 72, 72, 71, 71, 71, 71, 71, 71, 71, 71, 71, 71, 71, 71, 71, 71, 71, 71, 71, 71, 71, 71, 71, 71, 71, 71, 71, 71, 71, 71, 71, 71, 71, 71, 71, 71, 71, 71, 71, 71, 71, 71, 71, 71, 71, 71, 71, 71, 71, 71, 71, 71, 71, 71, 71, 71, 71, 71, 71, 71, 71, 71, 71, 71, 71, 71, 71, 71, 71, 71, 71, 71, 71, 71, 71, 71, 71, 71, 71, 71, 71, 71, 71, 71, 71, 71, 71, 71, 71, 71, 71, 71, 71, 71, 71, 71, 71, 71, 71, 71, 71, 71, 71, 71, 71, 71, 71, 71, 71, 71, 71, 71, 71, 71, 71, 71, 71, 71, 71, 71, 71, 71, 71, 71, 71, 71, 71, 71, 71, 71, 71, 71, 71, 71, 71, 71, 71, 71, 71, 71, 71, 71, 71, 71, 71, 71, 71, 71, 71, 71, 71, 71, 71, 71, 71, 71, 71, 71, 71, 71, 71, 71, 71, 71, 71, 71, 71, 71, 71, 71, 71, 71, 71, 71, 72, 72, 72, 72, 72, 72, 72, 72, 72, 72, 72, 72, 72, 72, 72, 72, 72, 72, 72, 72, 72, 72, 72, 72, 72, 72, 72, 72, 72, 72, 72, 72, 72, 72, 72, 72, 72, 72, 72, 72, 72, 72, 72, 72, 72, 72, 72, 72, 72, 72, 72, 72, 72, 72, 72, 72, 72, 72, 72, 72, 72, 72, 72, 72, 72, 72, 72, 72, 72, 72, 72, 72, 72, 72, 72, 72, 72, 72, 72, 72, 72, 72, 72, 72, 72, 72, 72, 72, 72, 72, 72, 72, 72, 72, 72, 72, 72, 72, 72, 72, 72, 72, 72, 72, 72, 72, 72, 72, 72, 72, 72, 72, 72, 72, 72, 72, 72, 72, 72, 72, 72, 72, 72, 72, 72, 72, 72, 72, 72, 72, 72, 72, 72, 72, 72, 72, 72, 72, 72, 72, 72, 72, 72, 72, 72, 72, 72, 72, 72, 72, 72, 72, 72, 72, 72, 72, 72, 72, 72, 72, 72, 72, 72, 72, 72, 72, 72, 72, 72, 72, 72, 72, 72, 72, 72, 72, 72, 72, 72, 72, 72, 72, 72, 72, 72, 72, 72, 72, 72, 72, 72, 72, 72, 72, 72, 72, 72, 72, 72, 72, 72, 72, 72, 72, 72, 72, 72, 72, 72, 72, 72, 72, 72, 72, 72, 72, 72, 72, 72, 72, 72, 72, 72, 72, 72, 72, 72, 72, 72, 72, 72, 72, 72, 72, 72, 72, 72, 72, 72, 72, 72, 72, 72, 72, 72, 72, 72, 72, 72, 72, 72, 72, 72, 72, 72, 72, 72, 72, 72, 72, 72, 72, 72, 72, 72, 72, 72, 72, 72, 72, 72, 72, 72, 72, 72, 72, 72, 72, 72, 72, 72, 72, 72, 72, 72, 72, 72, 72, 72, 72, 72, 72, 72, 72, 72, 72, 72, 72, 72, 72, 72, 72, 72, 72, 72, 72, 72, 72, 72, 72, 72, 72, 72, 72, 72, 72, 72, 72, 72, 72, 72, 72, 72, 72, 72, 72, 72, 72, 72, 72, 72, 72, 72, 72, 72, 72, 72, 72, 72, 72, 72, 72, 72, 72, 72, 72, 72, 72, 72, 72, 72, 72, 72, 72, 72, 72, 72, 72, 72, 72, 72, 72, 72, 72, 72, 72, 72, 72, 72, 72, 72, 72, 72, 72, 72, 72, 72, 72, 72, 72, 72, 72, 72, 72, 72, 72, 72, 72, 72, 72, 72, 72, 72, 72, 72, 72, 72, 72, 72, 72, 72, 72, 72, 72, 72, 72, 72, 72, 72, 72, 72, 72, 72, 72, 72, 72, 72, 72, 72, 72, 72, 72, 72, 72, 72, 72, 72, 72, 72, 72, 72, 72, 72, 72, 72, 72, 72, 72, 72, 72, 72, 72, 72, 72, 72, 72, 72, 72, 72, 72, 72, 72, 72, 72, 72, 72, 72, 72, 72, 72, 72, 72, 72, 72, 72, 72, 72, 72, 72, 72, 72, 72, 72, 72, 72, 72, 72, 72, 72, 72, 72, 72, 72, 72, 72, 72, 72, 72, 72, 72, 72, 72, 72, 72, 72, 72, 72, 72, 72, 72, 72, 72, 72, 72, 72, 72, 72, 72, 72, 72, 72, 72, 72, 72, 72, 72, 72, 72, 72, 72, 72, 72, 72, 72, 72, 72, 72, 72, 72, 72, 72, 72, 72, 72, 72, 72, 72, 72, 72, 72, 72, 72, 72, 72, 72, 72, 72, 72, 72, 72, 72, 72, 72, 72, 72, 72, 72, 72, 72, 72, 72, 72, 72, 72, 72, 72, 72, 72, 72, 72, 72, 72, 72, 72, 72, 72, 72, 72, 72, 72, 72, 72, 72, 72, 72, 72, 72, 72, 72, 72, 72, 72, 72, 72, 72, 72, 72, 72, 72, 72, 72, 72, 72, 72, 72, 72, 72, 72, 72, 72, 72, 72, 72, 72, 72, 72, 72, 72, 72, 72, 72, 72, 72, 72, 72, 72, 72, 72, 72, 72, 72, 72, 72, 72, 72, 72, 72, 72, 72, 72, 72, 72, 72, 72, 72, 72, 72, 72, 72, 72, 72, 72, 72, 72, 72, 72, 72, 72, 72, 72, 72, 72, 72, 72, 72, 72, 72, 72, 72, 72, 72, 72, 72, 72, 72, 72, 72, 72, 72, 72, 72, 72, 72, 72, 72, 72, 72, 72, 72, 73, 74, 75, 76, 77, 79, 82, 84, 88, 91, 96, 101, 109, 116, 124, 133, 142, 151, 161, 170, 180, 189, 198, 205, 212]
  in  "Triger Source":T3(ring)=enum."External"
  in  "Range Ch1":u32(ring)=3 items=["40mV", "100mV", "200mV", "400mV", "1 V", "2 V", "4 V"]
  in  "Range Ch2":u32(ring)=3 items=["40mV", "100mV", "200mV", "400mV", "1 V", "2 V", "4 V"]
  in  "Trig Slope":enum32{"Positive", "Negative"}(ring)
  in  "Trig Level":u32=144
  in  "Elevation Speed Factor":dbl=0.1
  in  "Lsr Interval (s)":dbl=2e-05
  out "VC Update ticks":u32=200
  in  "VCsamples":i32=1176
  in  "SaveLastSec":bool
  out "C-Scan Ticks":dbl=117600.0
  in  "clock rate (tick/sec)":i32=40000000
  out "ALAZAR9350":i32
  out "Trig interval":dbl=200.08003201280513
  out "vc_pt_sent":i32=805864
  out "AD_FIFO_SZ":i32=117600
  out "Ch1 Pt":i32=150528
  out "DAQ Trig #":i32=1176
  out "Laser Trig #":i32=1176 format="%#.6g"
  out "Aline Stop #":i32=35280000
  out "Y Steps Stop #":i32=480000
  in  "VC_EN":bool=TRUE
  out "DataQueue":refnum<queue>
  in  "save_rate":u32=40
  out "sum":dbl=117600.0
  in  "AuxVolt":i16=18500
  in  "AuxLength":u32
  out "file_ref":refnum<file>
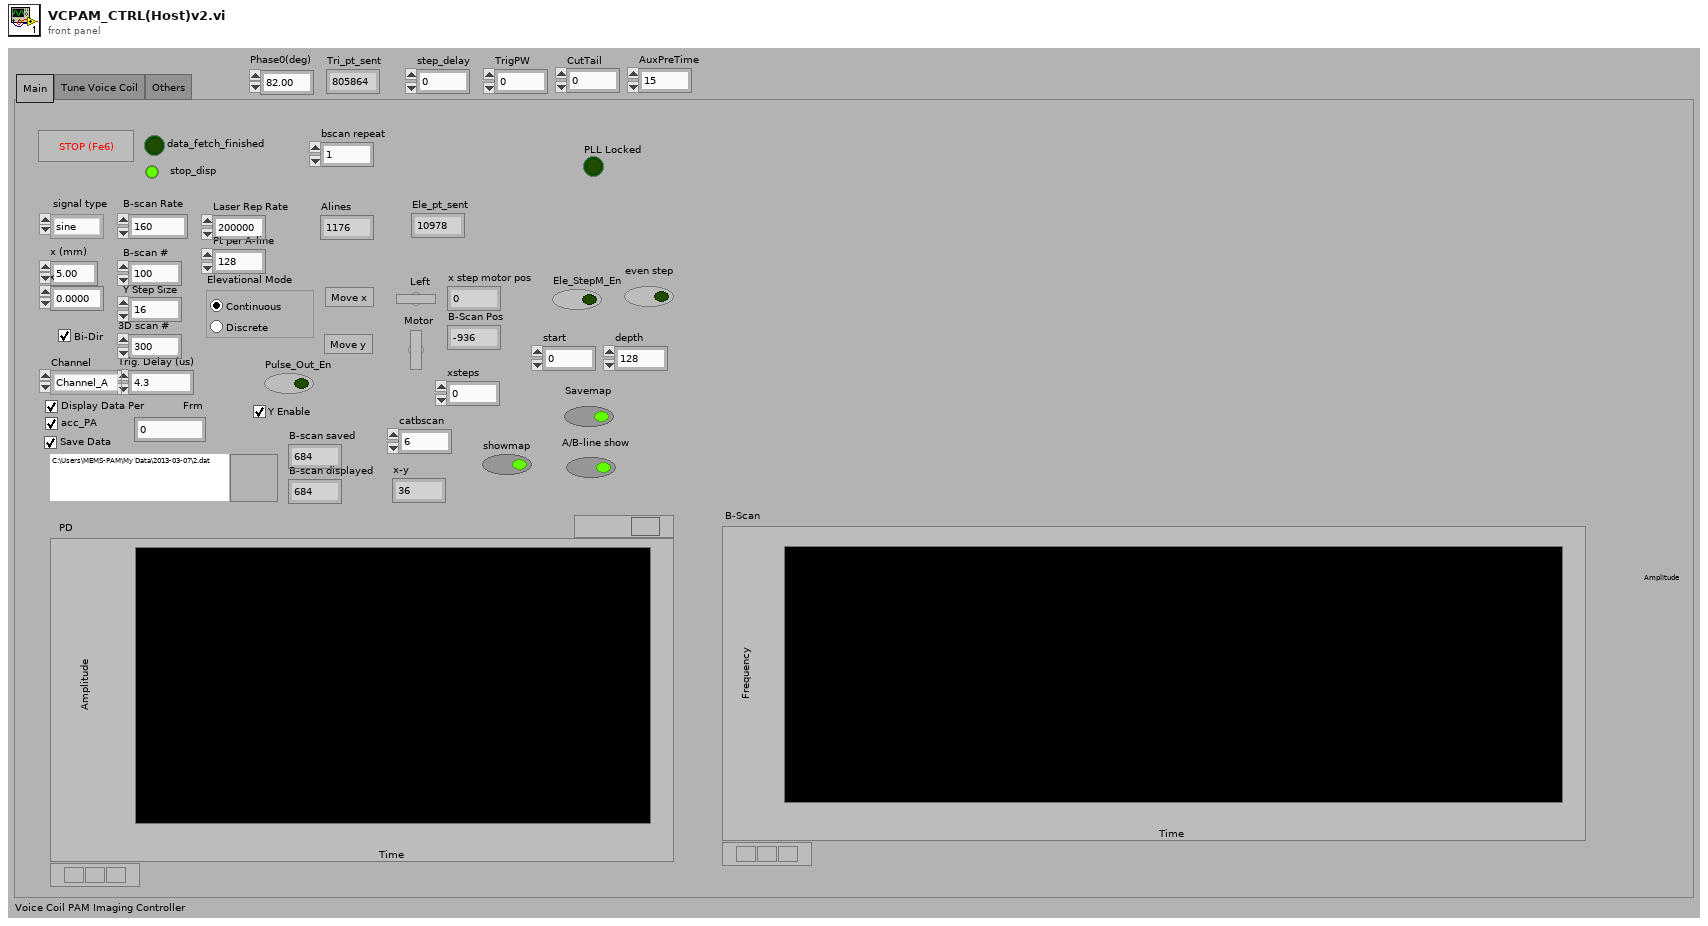
[diagram p1: front panel]
types:
  T1 = enum16{"sine", "cosine", "triangle", "square", "sawtooth", "increasing ramp", "decreasing ramp"}
  T2 = typedef "ATS_DMA_Channel.ctl" = enum16{"Channel_A", "Channel_B", "A & B"}
  T3 = enum32{"Chan_A", "Chan_B", "External", "Disable"}
  T4 = enum16{"big-endian, network order", "native, host order", "little-endian"}
  T5 = enum16{"open", "replace", "create", "open or create", "replace or create", "replace or create with confirmation"}
  T6 = typedef "nirio_resource_hc.ctl" = tag
  T7 = typedef "ATS_Async_Ctrl.ctl" = enum16{"SetupDMA", "StartCapture", "Get", "Get_Stream", "Abort", "Stop"}
  T8 = typedef "Device_Ctrl.ctl" = enum16{"Status", "About", "Arm", "ForceTrig", "Abort", "Initialize", "Init (NoPreset)", "Info", "Close", "Calibrate", "SetManually", "LED_ON", "LED_OFF"}
  T9 = typedef "ATS_Async_Status.ctl" = cluster{"Start DMA":bool, "StartCapture":bool, "Valid":bool, "Completed":bool, "InProgress":bool, "Timeout":bool, "Overflow":bool, "Error":bool}
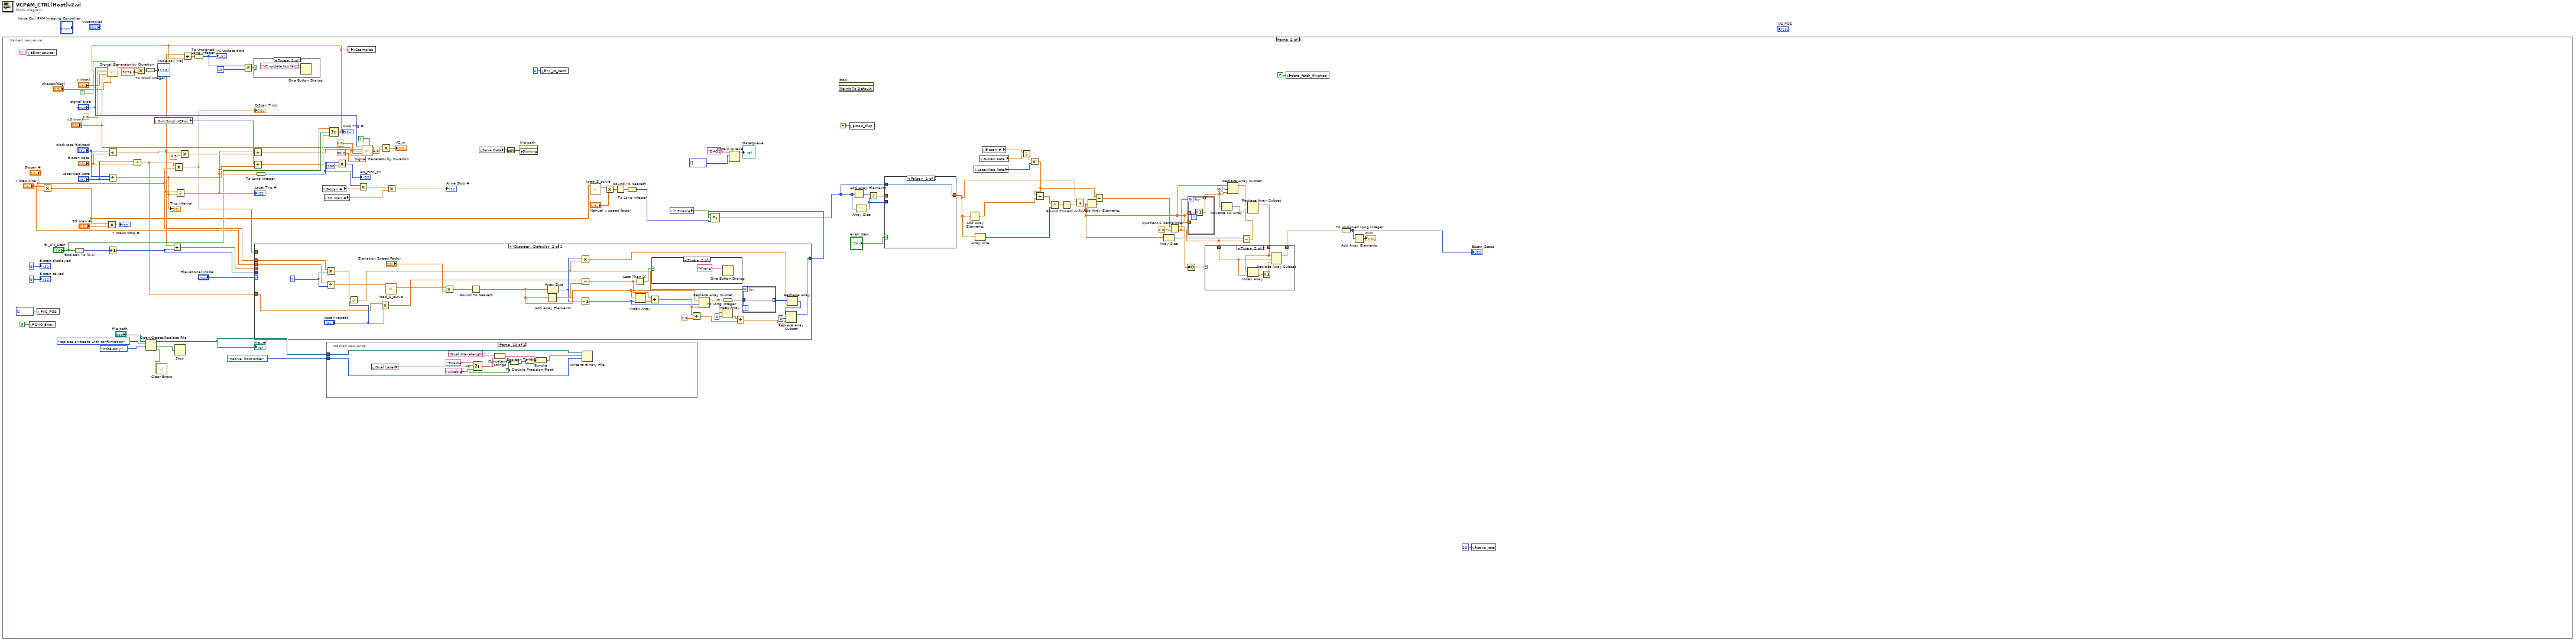
[diagram p0: block diagram]
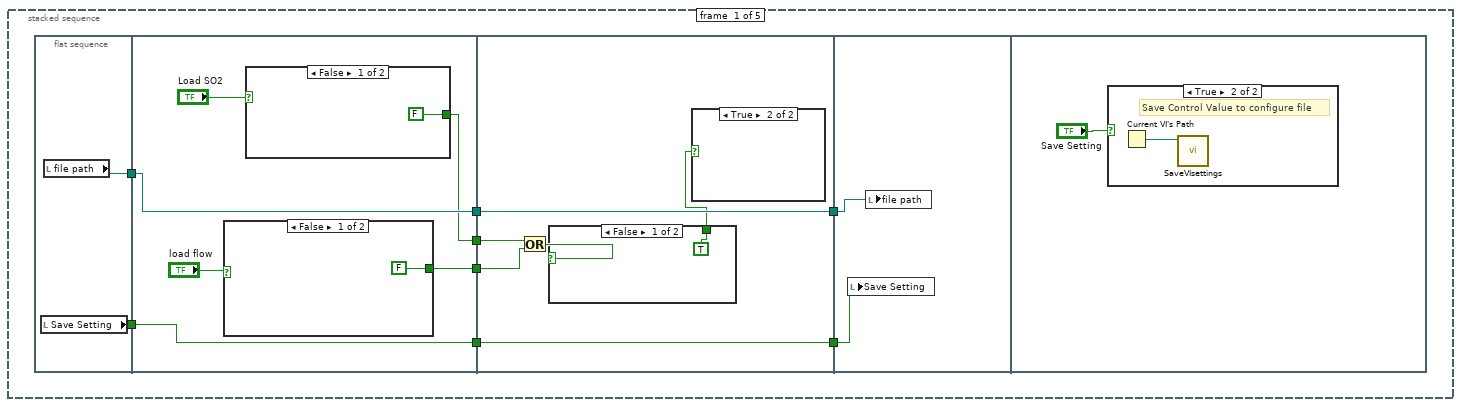
[diagram p2: hidden frame]
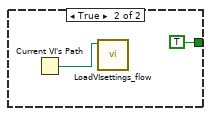
[diagram p3: hidden frame]
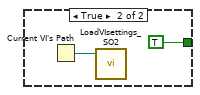
[diagram p4: hidden frame]
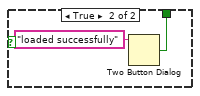
[diagram p5: hidden frame]
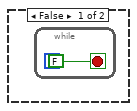
[diagram p6: hidden frame]
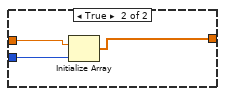
[diagram p9: hidden frame]
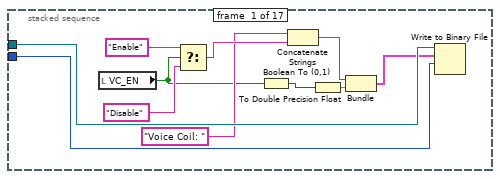
[diagram p11: hidden frame]
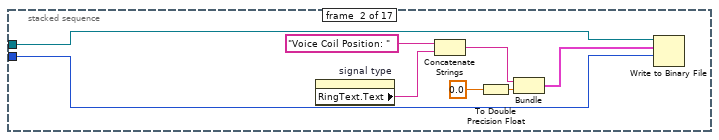
[diagram p12: hidden frame]
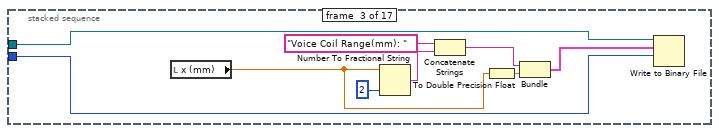
[diagram p13: hidden frame]
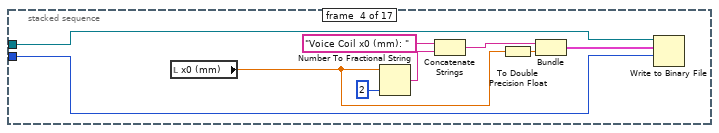
[diagram p14: hidden frame]
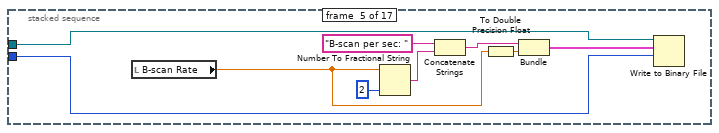
[diagram p15: hidden frame]
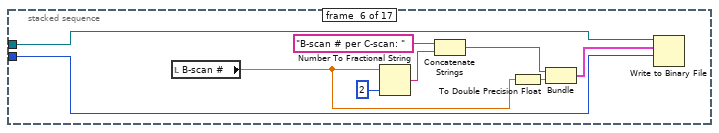
[diagram p16: hidden frame]
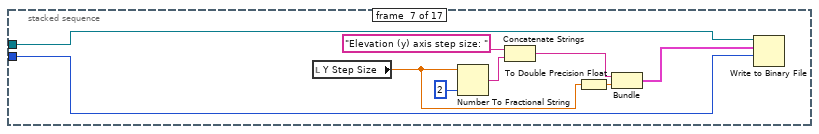
[diagram p17: hidden frame]
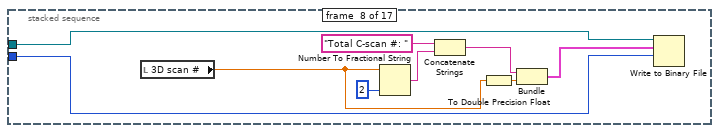
[diagram p18: hidden frame]
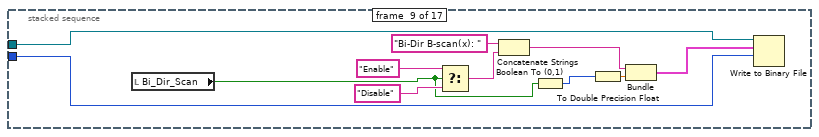
[diagram p19: hidden frame]
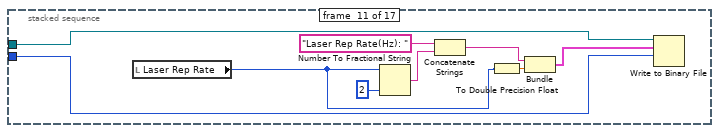
[diagram p20: hidden frame]
diagram:
  n1 = stacked-sequence {
    frame #0 {
      n2 = flat-sequence {
        tunnel: [w10] -> w8
        tunnel: [w9] -> w3
        tunnel: w8 -> [w14]
        tunnel: [w14] -> w6
        tunnel: [w13] -> w4
        tunnel: w3 -> [w13]
        tunnel: [w12] -> w2
        tunnel: [w11] -> w1
        tunnel: [w28] -> w7
        tunnel: w6 -> [w28]
        tunnel: [w27] -> w5
        tunnel: w4 -> [w27]
        tunnel: w2 -> [w26]
        tunnel: w1 -> [w25]
        tunnel: w7 -> [w34]
        tunnel: w5 -> [w33]
        frame #0 {
          n3 = local read "Save Setting"() -> (w9:bool)
          n4 = local read "file path"() -> (w10:path)
        }
        frame #1 {
          n5 = case shown="False" "load flow" {
            tunnel: [FALSE TRUE] -> w11
            frame False {
            }
            frame True {
              n6 = Current VI's Path() -> (path=w19:path)
              n7 = call "LoadVIsettings_flow.vi"("VI path"=w19) -> ()  [unwired: 11 in]
            }
          }
          n8 = case shown="False" "Load SO2" {
            tunnel: [FALSE TRUE] -> w12
            frame False {
            }
            frame True {
              n9 = Current VI's Path() -> (path=w22:path)
              n10 = call "LoadVIsettings_SO2.vi"("VI path"=w22) -> ()  [unwired: 11 in]
            }
          }
        }
        frame #2 {
          n11 = Or(x=w26, y=w25) -> (x .or. y?=w24:bool)
          n12 = case shown="False" w24 {
            tunnel: [TRUE ("T button?") w30] -> w23
            frame False {
            }
            frame True {
              n13 = Two Button Dialog(message="loaded successfully") -> (T button?=w30:bool)  [unwired: 2 in]
            }
          }
          n14 = case shown="True" w23 {
            frame False {
              n15 = while {
                stop <- FALSE stop-if-true
              }
            }
            frame True {
            }
          }
        }
        frame #3 {
          n16 = local write "Save Setting"(w33) -> ()
          n17 = local write "file path"(w34) -> ()
        }
        frame #4 {
          n18 = case shown="True" "Save Setting" {
            frame False {
            }
            frame True {
              # "Save Control Value to configure file"
              n19 = Current VI's Path() -> (path=w36:path)
              n20 = call "SaveVIsettings.vi"("path"=w36) -> ()  [unwired: 11 in]
            }
          }
        }
      }
    }
    frame #1 {
      w87 = 1.0 ("amplitude")
      n21 = local write "Error source"("" ("Error source")) -> ()
      n22 = local write "DAQ Error"(FALSE ("DAQ Error")) -> ()
      n23 = local write "VC_POS"(i16[] [] ("VC_POS")) -> ()
      n24 = Multiply(x="Y Step Size", y="B-scan #") -> (x*y=w95:dbl)
      n25 = Boolean To (0,1)(Boolean="Bi_Dir_Scan") -> (0, 1=w142:i16)
      n26 = Multiply(x=w95, y="3D scan #") -> (x*y=→"Y Steps Stop #":dbl)
      n27 = Divide(x="clock rate (tick/sec)", y="Laser Rep Rate") -> (x/y=w103:dbl)
      "Trig interval" <- w103
      n28 = Increment(x=w142) -> (x+1=w108:i16)
      n29 = Divide(x="clock rate (tick/sec)", y="B-scan Rate") -> (x/y=w67:dbl)
      n30 = Divide(x="Laser Rep Rate", y="B-scan Rate") -> (x/y=w37:dbl)
      n31 = Open/Create/Replace File(file path (use dialog)="file path", operation (0:open)=T5."replace or create with confirmation", access (0:read/write)=enum16{"read/write", "read-only", "write-only"}."write-only") -> (refnum out=w85:refnum<file>, cancelled=w84:bool, error out=w83:errorcluster)  [unwired: 1 in, 2 out]
      "file_ref" <- w85
      n32 = local read "DwnSmpl VCPos"() -> (w129:i32)
      n33 = call <vilib>:"Clear Errors.vi"("error in (no error)"=w83) -> ()  [unwired: 6 in, 1 out]
      n34 = Divide(x=w67, y=w108) -> (x/y=w143:dbl)
      n35 = Multiply(x=w37, y="B-scan #") -> (x*y=w70:dbl)
      "C-Scan Ticks" <- w70
      n36 = Stop(stop? (T)=w84) -> ()
      n37 = Divide(x=w67, y=w103) -> (x/y=w106:dbl)
      "Laser Trig #" <- w106
      n38 = Multiply(x=w67, y=0.5 ("frequency")) -> (x*y=w140:dbl)
      n39 = Divide(x=w106, y=w129) -> (x/y=w127:dbl)
      n40 = Divide(x=w140, y=w103) -> (x/y=w138:dbl)
      n41 = case shown="\"Discrete\", Default" "Elevational Mode" {
        tunnel: [w329 w336] -> w92
        tunnel: "Y Step Size" -> [w328 w348]
        tunnel: w70 -> [w326 _]
        tunnel: w143 -> [_ _]
        tunnel: "B-scan #" -> [w325 w346]
        tunnel: w108 -> [_ _]
        tunnel: w37 -> [_ w330]
        frame "Continuous" {
          n42 = Multiply(x=w328, y=w325) -> (x*y=w327:dbl)
          n43 = call "load_S_curve.vi"("samples"=w326, "pulses"=w327) -> ("S Curve"=w329:i32[])  [unwired: 8 in, 1 out]
        }
        frame "Discrete", Default {
          w331 = 1
          n44 = Multiply(x=w346, y=w331) -> (x*y=w333:dbl)
          n45 = Divide(x=w348, y=w331) -> (x/y=w347:dbl)
          n46 = Divide(x=w333, y="bscan repeat") -> (x/y=w332:dbl)
          n47 = Multiply(x=w330, y="bscan repeat") -> (x*y=w335:dbl)
          n48 = call "load_S_curve.vi"("pulses"=w347) -> ("Raw S Curve"=w361:dbl[])  [unwired: 9 in, 1 out]
          n49 = Multiply(x=w361, y="Elevation Speed Factor") -> (x*y=w360:dbl[])
          n50 = Round To Nearest(number=w360) -> (nearest integer value=w352:dbl[])
          n51 = Add Array Elements(numeric array=w352) -> (sum=w359:dbl)
          n52 = Array Size(array=w352) -> (size(s)=w354:i32)
          n53 = Multiply(x=w354, y=w332) -> (x*y=w353:dbl)
          n54 = Subtract(x=w335, y=w359) -> (x-y=w351:dbl)
          n55 = Decrement(x=w354) -> (x-1=w357:i32)
          n56 = Less Than 0?(x=w351) -> (x < 0?=w350:bool)
          n57 = Index Array(array=w352, index=w357) -> (element=w358:dbl)
          n58 = Add(x=w351, y=w358) -> (x+y=w345:dbl)
          n59 = case shown="True" w350 {
            frame False {
            }
            frame True {
              n60 = One Button Dialog(message="Wrong") -> ()  [unwired: 1 in, 1 out]
            }
          }
          n61 = Divide(x=w345, y=2.0) -> (x/y=w341:dbl)
          n62 = Replace Array Subset(array=w352, new element=w345, index=w357) -> (w343:dbl[])
          n63 = Index Array(array=w343, index=0) -> (element=w340:dbl)
          n64 = To Long Integer(number=w343) -> (32bit integer=w356:i32[])
          n65 = Add(x=w340, y=w341) -> (x+y=w337:dbl)
          n66 = for {
            N: w332 -> [_]
            tunnel: w356 -> [w363]
            tunnel: [w363] -> w355 mode=indexing
          }
          n67 = Reshape Array(w355, w353) -> (w339:i32[])
          n68 = Replace Array Subset(array=w339, new element=w337, index=0) -> (w336:i32[])
        }
      }
      n69 = To Long Integer(number=w106) -> (32bit integer=w130:i32)
      n70 = local read "B-scan #"() -> (w107:dbl)
      n71 = local read "3D scan #"() -> (w136:dbl)
      n72 = stacked-sequence {
        tunnel: w85 -> [w171 w180 w189 w198 w204 w212 w223 w231 w245 w254 w262 w271 w279 w292 w302 w317 w323]
        tunnel: T4."native, host order" ("byte order (0:big-endian, network order)") -> [w172 w179 w188 w197 w203 w213 w222 w230 w244 w253 w261 w270 w280 w291 w301 w316 w324]
        frame #0 {
          n73 = local read "VC_EN"() -> (w162:bool)
          n74 = Select(t="Enable", s=w162, f="Disable") -> (s? t:f=w168:string)
          n75 = Boolean To (0,1)(Boolean=w162) -> (0, 1=w163:i16)
          n76 = Concatenate Strings("Voice Coil: " ("string"), w168) -> (w165:string)
          n77 = To Double Precision Float(number=w163) -> (double precision float=w166:dbl)
          n78 = Bundle(w165, w166) -> (w164:cluster{string, dbl})  [unwired: 1 in]
          n79 = Write to Binary File(file (use dialog)=w171, data=w164, 9:w172) -> ()  [unwired: 3 in, 3 out]
        }
        frame #1 {
          n80 = property on="signal type" class="Enum (strict)"() -> ("RingText.Text"=w178:string)  [unwired: 2 in, 2 out]
          n81 = Concatenate Strings("Voice Coil Position: " ("string"), w178) -> (w174:string)
          n82 = To Double Precision Float(number=0.0) -> (double precision float=w176:dbl)
          n83 = Bundle(w174, w176) -> (w175:cluster{string, dbl})  [unwired: 1 in]
          n84 = Write to Binary File(file (use dialog)=w180, data=w175, 9:w179) -> ()  [unwired: 2 in, 4 out]
        }
        frame #2 {
          n85 = local read "x (mm)"() -> (w181:dbl)
          n86 = Number To Fractional String(number=w181, precision (6)=i16 2) -> (F-format string=w186:string)  [unwired: 2 in]
          n87 = Concatenate Strings("Voice Coil Range(mm): " ("string"), w186) -> (w182:string)
          n88 = To Double Precision Float(number=w181) -> (double precision float=w184:dbl)
          n89 = Bundle(w182, w184) -> (w183:cluster{string, dbl})  [unwired: 1 in]
          n90 = Write to Binary File(file (use dialog)=w189, data=w183, 9:w188) -> ()  [unwired: 2 in, 4 out]
        }
        frame #3 {
          n91 = local read "x0 (mm)"() -> (w190:dbl)
          n92 = Number To Fractional String(number=w190, precision (6)=i16 2) -> (F-format string=w195:string)  [unwired: 2 in]
          n93 = Concatenate Strings("Voice Coil x0 (mm): " ("string"), w195) -> (w191:string)
          n94 = To Double Precision Float(number=w190) -> (double precision float=w193:dbl)
          n95 = Bundle(w191, w193) -> (w192:cluster{string, dbl})  [unwired: 1 in]
          n96 = Write to Binary File(file (use dialog)=w198, data=w192, 9:w197) -> ()  [unwired: 2 in, 4 out]
        }
        frame #4 {
          n97 = local read "B-scan Rate"() -> (w199:dbl)
          n98 = Number To Fractional String(number=w199, precision (6)=i16 2) -> (F-format string=w206:string)  [unwired: 2 in]
          n99 = Concatenate Strings("B-scan per sec: " ("string"), w206) -> (w200:string)
          n100 = To Double Precision Float(number=w199) -> (double precision float=w202:dbl)
          n101 = Bundle(w200, w202) -> (w201:cluster{string, dbl})  [unwired: 1 in]
          n102 = Write to Binary File(file (use dialog)=w204, data=w201, 9:w203) -> ()  [unwired: 2 in, 4 out]
        }
        frame #5 {
          n103 = local read "B-scan #"() -> (w208:dbl)
          n104 = Number To Fractional String(number=w208, precision (6)=i16 2) -> (F-format string=w215:string)  [unwired: 2 in]
          n105 = Concatenate Strings("B-scan # per C-scan: " ("string"), w215) -> (w209:string)
          n106 = To Double Precision Float(number=w208) -> (double precision float=w211:dbl)
          n107 = Bundle(w209, w211) -> (w210:cluster{string, dbl})  [unwired: 1 in]
          n108 = Write to Binary File(file (use dialog)=w212, data=w210, 9:w213) -> ()  [unwired: 2 in, 4 out]
        }
        frame #6 {
          n109 = local read "Y Step Size"() -> (w217:dbl)
          n110 = Number To Fractional String(number=w217, precision (6)=i16 2) -> (F-format string=w221:string)  [unwired: 2 in]
          n111 = Concatenate Strings("Elevation (y) axis step size: " ("string"), w221) -> (w218:string)
          n112 = To Double Precision Float(number=w217) -> (double precision float=w220:dbl)
          n113 = Bundle(w218, w220) -> (w219:cluster{string, dbl})  [unwired: 1 in]
          n114 = Write to Binary File(file (use dialog)=w223, data=w219, 9:w222) -> ()  [unwired: 2 in, 4 out]
        }
        frame #7 {
          n115 = local read "3D scan #"() -> (w226:dbl)
          n116 = Number To Fractional String(number=w226, precision (6)=i16 2) -> (F-format string=w233:string)  [unwired: 2 in]
          n117 = Concatenate Strings("Total C-scan #: " ("string"), w233) -> (w227:string)
          n118 = To Double Precision Float(number=w226) -> (double precision float=w229:dbl)
          n119 = Bundle(w227, w229) -> (w228:cluster{string, dbl})  [unwired: 1 in]
          n120 = Write to Binary File(file (use dialog)=w231, data=w228, 9:w230) -> ()  [unwired: 2 in, 4 out]
        }
        frame #8 {
          n121 = local read "Bi_Dir_Scan"() -> (w235:bool)
          n122 = Select(t="Enable", s=w235, f="Disable") -> (s? t:f=w240:string)
          n123 = Concatenate Strings("Bi-Dir B-scan(x): " ("string"), w240) -> (w238:string)
          n124 = Boolean To (0,1)(Boolean=w235) -> (0, 1=w236:i16)
          n125 = To Double Precision Float(number=w236) -> (double precision float=w239:dbl)
          n126 = Bundle(w238, w239) -> (w237:cluster{string, dbl})  [unwired: 1 in]
          n127 = Write to Binary File(file (use dialog)=w245, data=w237, 9:w244) -> ()  [unwired: 2 in, 4 out]
        }
        frame #9 {
          n128 = local read "Dual Laser"() -> (w247:bool)
          n129 = Select(t="Enable", s=w247, f="Disable") -> (s? t:f=w251:string)
          n130 = Concatenate Strings("Dual Wavelength:" ("string"), w251) -> (w248:string)
          n131 = Boolean To (0,1)(Boolean=w247) -> (0, 1=w246:i16)
          n132 = To Double Precision Float(number=w246) -> (double precision float=w250:dbl)
          n133 = Bundle(w248, w250) -> (w249:cluster{string, dbl})  [unwired: 1 in]
          n134 = Write to Binary File(file (use dialog)=w254, data=w249, 9:w253) -> ()  [unwired: 2 in, 4 out]
        }
        frame #10 {
          n135 = local read "Laser Rep Rate"() -> (w257:u32)
          n136 = Number To Fractional String(number=w257, precision (6)=i16 2) -> (F-format string=w264:string)  [unwired: 2 in]
          n137 = Concatenate Strings("Laser Rep Rate(Hz): " ("string"), w264) -> (w258:string)
          n138 = To Double Precision Float(number=w257) -> (double precision float=w260:dbl)
          n139 = Bundle(w258, w260) -> (w259:cluster{string, dbl})  [unwired: 1 in]
          n140 = Write to Binary File(file (use dialog)=w262, data=w259, 9:w261) -> ()  [unwired: 2 in, 4 out]
        }
        frame #11 {
          n141 = local read "Lsr Interval (s)"() -> (w266:dbl)
          n142 = Number To Fractional String(number=w266, precision (6)=i16 8) -> (F-format string=w273:string)  [unwired: 2 in]
          n143 = Concatenate Strings("Laser time interval: " ("string"), w273) -> (w267:string)
          n144 = To Double Precision Float(number=w266) -> (double precision float=w269:dbl)
          n145 = Bundle(w267, w269) -> (w268:cluster{string, dbl})  [unwired: 1 in]
          n146 = Write to Binary File(file (use dialog)=w271, data=w268, 9:w270) -> ()  [unwired: 2 in, 4 out]
        }
        frame #12 {
          n147 = local read "Pt per A-line"() -> (w275:i32)
          n148 = Number To Fractional String(number=w275, precision (6)=i16 2) -> (F-format string=w282:string)  [unwired: 2 in]
          n149 = Concatenate Strings("Pt per Aline: " ("string"), w282) -> (w276:string)
          n150 = To Double Precision Float(number=w275) -> (double precision float=w278:dbl)
          n151 = Bundle(w276, w278) -> (w277:cluster{string, dbl})  [unwired: 1 in]
          n152 = Write to Binary File(file (use dialog)=w279, data=w277, 9:w280) -> ()  [unwired: 2 in, 4 out]
        }
        frame #13 {
          n153 = local read "Elevational Mode"() -> (w284:enum32{"Continuous", "Discrete"})
          n154 = Equal?(x=w284, y=enum32{"Continuous", "Discrete"}."Continuous" ("Elevational Mode")) -> (x = y?=w289:bool)
          n155 = Select(t="Continuous", s=w289, f="Discrete") -> (s? t:f=w293:string)
          n156 = Concatenate Strings("Elevational (y) Scan Mode: " ("string"), w293) -> (w285:string)
          n157 = To Double Precision Float(number=w284) -> (double precision float=w287:dbl)
          n158 = Bundle(w285, w287) -> (w286:cluster{string, dbl})  [unwired: 1 in]
          n159 = Write to Binary File(file (use dialog)=w292, data=w286, 9:w291) -> ()  [unwired: 2 in, 4 out]
        }
        frame #14 {
          n160 = local read "Ele_Ini_Dir"() -> (w297:bool)
          n161 = Select(t="Towards Motor", s=w297, f="Away Motor") -> (s? t:f=w303:string)
          n162 = Concatenate Strings("Y Direction:" ("string"), w303) -> (w299:string)
          n163 = Boolean To (0,1)(Boolean=w297) -> (0, 1=w296:i16)
          n164 = To Double Precision Float(number=w296) -> (double precision float=w300:dbl)
          n165 = Bundle(w299, w300) -> (w298:cluster{string, dbl})  [unwired: 1 in]
          n166 = Write to Binary File(file (use dialog)=w302, data=w298, 9:w301) -> ()  [unwired: 2 in, 4 out]
        }
        frame #15 {
          n167 = Build Array("CH_A", "CH_B", "CH_A_B") -> (w312:string[])
          n168 = local read "Channel"() -> (w307:T2)
          n169 = Index Array(array=w312, index=w307) -> (element=w311:string)
          n170 = Concatenate Strings("Chan: " ("string"), w311) -> (w309:string)
          n171 = To Double Precision Float(number=w307) -> (double precision float=w310:dbl)
          n172 = Bundle(w309, w310) -> (w308:cluster{string, dbl})  [unwired: 1 in]
          n173 = Write to Binary File(file (use dialog)=w317, data=w308, 9:w316) -> ()  [unwired: 2 in, 4 out]
        }
        frame #16 {
          n174 = To Double Precision Float(number=0.0) -> (double precision float=w320:dbl)
          n175 = Bundle("/*END*/", w320) -> (w321:cluster{string, dbl})  [unwired: 1 in]
          n176 = Write to Binary File(file (use dialog)=w323, data=w321, 9:w324) -> ()  [unwired: 2 in, 4 out]
        }
      }
      n177 = Select(t=w106, s="Bi_Dir_Scan", f=w138) -> (s? t:f=w72:dbl)
      "DAQ Trig #" <- w72
      n178 = call <vilib>:"Signal Generator by Duration.vi"("signal type"="signal type", "reset phase"=TRUE, "# of samples"=w72, "frequency"=1.0, "amplitude"="x (mm)", "dc offset"="x0 (mm)", "phase in"="Phase0(deg)") -> ("signal"=w88:dbl[])  [unwired: 5 in, 3 out]
      n179 = Multiply(x=w88, y=3276.8 ("frequency")) -> (x*y=w146:dbl[])
      n180 = To Word Integer(number=w146) -> (16bit integer=→"Vocie-coil Traj":i16[])
      n181 = Divide(x=w67, y=w72) -> (x/y=w148:dbl)
      n182 = To Unsigned Long Integer(number=w148) -> (unsigned 32bit integer=w102:u32)
      "VC Update ticks" <- w102
      n183 = Less Or Equal?(x=w102, y=u32 40) -> (x <= y?=w100:bool)
      n184 = case shown="True" w100 {
        frame False {
        }
        frame True {
          n185 = One Button Dialog(message="VC update too fast!") -> ()  [unwired: 1 in, 1 out]
        }
      }
      n186 = Multiply(x=w130, y=100 ("frequency")) -> (x*y=→"AD_FIFO_SZ":i32)
      n187 = local write "VCsamples"(w72) -> ()
      n188 = Multiply(x=w130, y=w107) -> (x*y=w137:dbl)
      n189 = call <vilib>:"Signal Generator by Duration.vi"("signal type"="signal type", "reset phase"=TRUE, "# of samples"=w127, "frequency"=w87, "amplitude"=w87, "dc offset"="x0 (mm)", "phase in"=90.0) -> ("signal"=w122:dbl[])  [unwired: 5 in, 3 out]
      n190 = Multiply(x=w122, y=1.0 ("phase in")) -> (x*y=→"VC_In":dbl[])
      n191 = Multiply(x=w137, y=w136) -> (x*y=→"Aline Stop #":dbl)
      n192 = local read "Save Data"() -> (w89:bool)
      n193 = Not(x=w89) -> (.not. x?=w90:bool)
      n194 = property on="file path" class="Path"("Blinking"=w90) -> ()  [unwired: 2 in, 2 out]
      n195 = local write "Tri_pt_sent"(0 ("Tri_pt_sent")) -> ()
      n196 = call "load_S_curve.vi"("pulses"=w95) -> ("Raw S Curve"=w98:dbl[])  [unwired: 9 in, 1 out]
      n197 = Multiply(x=w98, y="Manual y speed factor") -> (x*y=w97:dbl[])
      n198 = Round To Nearest(number=w97) -> (nearest integer value=w96:dbl[])
      n199 = To Long Integer(number=w96) -> (32bit integer=w91:i32[])
      n200 = local read "Y Enable"() -> (w93:bool)
      n201 = Select(t=w92, s=w93, f=w91) -> (s? t:f=w78:i32[])
      n202 = Obtain Queue(name (unnamed)="DAQ1", element data type=u16[] [] ("Buffer")) -> (queue out=→"DataQueue":refnum<queue>)  [unwired: 3 in, 2 out]
      n203 = invoke on="stop" class="Bool" method="Reinit To Default"() -> ()  [unwired: 3 in, 3 out]
      n204 = local write "stop_disp"(FALSE ("stop_disp")) -> ()
      n205 = Add Array Elements(numeric array=w78) -> (sum=w81:i32)
      n206 = Array Size(array=w78) -> (size(s)=w79:i32)
      n207 = Divide(x=w81, y=w79) -> (x/y=w80:dbl)
      n208 = case shown="False" "even step" {
        tunnel: w80 -> [_ w160]
        tunnel: w79 -> [_ w159]
        tunnel: [w157 w158] -> w52
        tunnel: w78 -> [w157 _]
        frame False {
        }
        frame True {
          n209 = Initialize Array(w160, w159) -> (w158:dbl[])
        }
      }
      n210 = Add Array Elements(numeric array=w52) -> (sum=w61:dbl)
      n211 = local read "Laser Rep Rate"() -> (w62:u32)
      n212 = Array Size(array=w52) -> (size(s)=w59:i32)
      n213 = local read "B-scan Rate"() -> (w64:dbl)
      n214 = local read "B-scan #"() -> (w65:dbl)
      n215 = Divide(x=w65, y=w64) -> (x/y=w63:dbl)
      n216 = Multiply(x=w63, y=w62) -> (x*y=w55:dbl)
      n217 = Subtract(x=w55, y=w61) -> (x-y=w60:dbl)
      n218 = Divide(x=w60, y=w59) -> (x/y=w58:dbl)
      n219 = Round Toward -Infinity(1:w58) -> (0:w57:dbl)
      n220 = Add(x=w52, y=w57) -> (x+y=w56:dbl[])
      n221 = Add Array Elements(numeric array=w56) -> (sum=w54:dbl)
      n222 = Subtract(x=w55, y=w54) -> (x-y=w53:dbl)
      n223 = Array Size(array=w56) -> (size(s)=w47:i32)
      n224 = Quotient & Remainder(x=w53, y=2.0) -> (x-y*floor(x/y)=w44:dbl, floor(x/y)=w41:dbl)
      n225 = Not Equal To 0?(x=w44) -> (x != 0?=w43:bool)
      n226 = for {
        N: w41 -> [_]
        tunnel: w56 -> [w156] mode=indexing
        tunnel: [w155] -> w49 mode=indexing
        tunnel: w56 -> [_]
        n227 = Increment(x=w156) -> (x+1=w155:dbl)
      }
      n228 = Reverse 1D Array(array=w49) -> (reversed array=w45:dbl[])
      n229 = Replace Array Subset(array=w56, new element=w49, index=0) -> (w48:dbl[])
      n230 = Subtract(x=w47, y=w41) -> (x-y=w46:dbl)
      n231 = Replace Array Subset(array=w48, new element=w45, index=w46) -> (w42:dbl[])
      n232 = case shown="True" w43 {
        tunnel: w42 -> [w149 w153]
        tunnel: [w149 w154] -> w40
        tunnel: w41 -> [_ w152]
        frame False {
        }
        frame True {
          n233 = Index Array(array=w153, index=w152) -> (element=w151:dbl)
          n234 = Increment(x=w151) -> (x+1=w150:dbl)
          n235 = Replace Array Subset(array=w153, new element=w150, index=w152) -> (w154:dbl[])
        }
      }
      n236 = local write "data_fetch_finished"(FALSE ("data_fetch_finished")) -> ()
      n237 = To Unsigned Long Integer(number=w40) -> (unsigned 32bit integer=w38:u32[])
      "Bscan_Steps" <- w38
      n238 = Add Array Elements(numeric array=w38) -> (sum=→"sum":u32)
      n239 = local write "save_rate"(u32 10 ("save_rate")) -> ()
      "B-scan saved" <- 0 ("saved bscan")
      "B-scan displayed" <- 0 ("saved bscan 2")
    }
    frame #2 {
      n240 = local read "VCsamples"() -> (w426:i32)
      n241 = local read "Bscan_Steps"() -> (w389:u32[])
      n242 = xnode "FPGA Open VI Reference"("resource name"=T6 "RIO0") -> ("FPGA VI Reference Out"=w439:refnum<k20>, "error out"=w440:errorcluster)  [unwired: 1 in]
      n243 = local read "clock rate (tick/sec)"() -> (w398:i32)
      n244 = xnode "Invoke Method"("FPGA VI Reference In"=w439, "error in"=w440) -> ("FPGA VI Reference Out"=w441:refnum<k20>, "error out"=w442:errorcluster)
      n245 = Multiply(x=w426, y=2) -> (x*y=w425:i32)
      n246 = xnode "Invoke Method"("FPGA VI Reference In"=w441, "error in"=w442, "Depth"=w425) -> ("FPGA VI Reference Out"=w378:refnum<k20>, "error out"=w379:errorcluster)
      n247 = Array Size(array=w389) -> (size(s)=w388:i32)
      n248 = Multiply(x=2, y=w388) -> (x*y=w418:i32)
      n249 = xnode "Invoke Method"("FPGA VI Reference In"=w378, "error in"=w379, "Depth"=w418) -> ("FPGA VI Reference Out"=w422:refnum<k20>, "error out"=w423:errorcluster)
      n250 = local read "Y Enable"() -> (w405:bool)
      n251 = local read "DAQ Trig #"() -> (w374:i32)
      n252 = case shown="True" w405 {
        tunnel: w423 -> [w564 w570]
        tunnel: w422 -> [w565 w569]
        tunnel: [w565 w568] -> w421
        tunnel: [w564 w567] -> w420
        tunnel: w389 -> [_ w566]
        frame False {
        }
        frame True {
          n253 = xnode "Invoke Method"("FPGA VI Reference In"=w569, "error in"=w570, "Data"=w566) -> ("FPGA VI Reference Out"=w568:refnum<k20>, "error out"=w567:errorcluster)  [unwired: 1 in, 1 out]
        }
      }
      n254 = local read "Vocie-coil Traj"() -> (w391:i16[])
      n255 = local read "Laser Rep Rate"() -> (w399:u32)
      n256 = Insert Into Array(array=w391, new element=w391) -> ()  [unwired: 1 in, 1 out]
      n257 = Divide(x=w398, y=w399) -> (x/y=w396:dbl)
      n258 = Multiply(x=w398, y="Lsr Interval (s)") -> (x*y=w395:dbl)
      n259 = xnode "Invoke Method"("FPGA VI Reference In"=w421, "error in"=w420, "Data"=w391) -> ("FPGA VI Reference Out"=w416:refnum<k20>, "error out"=w443:errorcluster)  [unwired: 1 in, 1 out]
      n260 = local read "Aline Stop #"() -> (w365:i32)
      n261 = local read "x step motor pos"() -> (w407:i32)
      n262 = local read "VC Update ticks"() -> (w419:u32)
      n263 = Not(x="Ele_Ini_Dir") -> (.not. x?=w392:bool)
      n264 = To Unsigned Long Integer(number=w396) -> ()  [unwired: 1 out]
      n265 = To Unsigned Long Integer(number=w395) -> (unsigned 32bit integer=w394:u32)
      n266 = local read "Y Steps Stop #"() -> (w406:i32)
      n267 = local read "Laser Trig #"() -> (w415:i32)
      n268 = local read "VCsamples"() -> (w390:i32)
      n269 = local read "B-Scan Pos"() -> (w408:i32)
      n270 = Add(x=w365, y="CutTail") -> (x+y=w364:dbl)
      n271 = local read "Left"() -> (w386:bool)
      n272 = xnode "Read/Write Control"("FPGA VI Reference In"=w416, "error in"=w443, "FIFO_Timeout"=40000, "VC_Update_Time"=w419, "VC_EN"="VC_EN", "Ele_StepM_En"=FALSE ("Bscan_StepM_En"), "Bscan_StepM_En"="Ele_StepM_En", "stop"=FALSE, "Ele_Ini_Dir"=w392, "Ele_total_steps"=w388, "DualWavelengthInterval"=w394, "DAQ Trig #"=w374, "Laser Trig #"=w415, "B-scan Stop Steps"=w406, "Scan"="Y Enable", "Aline Stop #"=w364, "B-Scan Pos"=w408, "x step motor pos"=w407, "start_scan"=FALSE, "Trig#todld"=w374, "VC_pt_in_fifo"=w390, "YStpMPlsInFifo"=w388, "Pulse_Out_En"="Pulse_Out_En", "B-scan Dir"=w386, "xsteps"="xsteps", "x_scan"=FALSE, "pls_V"=i16 32000, "PW"=u8 80, "TrigPW"="TrigPW", "AuxVolt"="AuxVolt", "AuxPreTime"="AuxPreTime", "catbscan"="catbscan") -> ("FPGA VI Reference Out"=w437:refnum<k20>, "error out"=w427:errorcluster)
      n273 = flat-sequence {
        tunnel: w437 -> [w534]
        tunnel: w427 -> [w531]
        tunnel: [w533] -> w401
        tunnel: [w532] -> w400
        tunnel: w401 -> [w537]
        tunnel: w400 -> [w536]
        tunnel: [w537] -> w373
        tunnel: [w536] -> w371
        tunnel: w373 -> [w558]
        tunnel: [w558] -> w372
        tunnel: w371 -> [w557]
        tunnel: [w557] -> w370
        tunnel: [w560] -> w435
        tunnel: [w562] -> w436
        tunnel: w372 -> [w563]
        tunnel: w370 -> [w561]
        frame #0 {
          n274 = xnode "Invoke Method"("FPGA VI Reference In"=w534, "error in"=w531) -> ("FPGA VI Reference Out"=w533:refnum<k20>, "error out"=w532:errorcluster)  [unwired: 1 in]
          n275 = Wait Until Next ms Multiple(millisecond multiple=u32 2) -> ()  [unwired: 1 out]
        }
        frame #1 {
          n276 = local read "acc_PA"() -> (w535:bool)
          n277 = case shown="True" w535 {
            frame False {
            }
            frame True {
              n278 = local read "DAQ Trig #"() -> (w539:i32)
              "Alines" <- w539
              n279 = local read "B-scan #"() -> (w541:dbl)
              n280 = local read "catbscan"() -> (w540:i16)
              n281 = Multiply(x="Pt per A-line", y=w539) -> (x*y=→"Ch1 Pt":i32)
              n282 = Initialize Array(0.0 ("element"), w539, w541) -> (→"MAP":dbl[][])
              n283 = Multiply(x=w539, y=w540) -> (x*y=w538:i32)
              n284 = call "Digitizer_initialization.vi"("Device"=0, "Triger Source"="Triger Source", "RecordLength"="Pt per A-line", "9350_Range 2"="Range Ch2", "9350_Range"="Range Ch1", "Channel"="Channel", "Trig. Delay (us)"="Trig. Delay (us)", "Level"="Trig Level", "Slope"="Trig Slope", "Rec/Buf"=w538) -> ("PLL Locked"=→"PLL Locked":bool, "DeviceOut"=→"ALAZAR9350":i32)  [unwired: 3 in, 1 out]
            }
          }
        }
        frame #2 {
          n285 = Wait Until Next ms Multiple(millisecond multiple=u32 100) -> ()  [unwired: 1 out]
        }
        frame #3 {
          n286 = xnode "Read/Write Control"("FPGA VI Reference In"=w563, "error in"=w561, "start_scan"=TRUE) -> ("FPGA VI Reference Out"=w562:refnum<k20>, "error out"=w560:errorcluster)
        }
      }
      n287 = Tick Count (ms)() -> (millisecond timer value=w403:u32)
      n288 = while {
        tunnel: w436 -> [w590]
        shift-right: [w587] -> w433
        shift-left: w435 -> [w589]
        tunnel: [w588] -> w434
        shift-right: [w585] -> _
        shift-left: i32[] [] -> [w576]
        shift-right: [w579] -> _
        shift-left: w403 -> [w571]
        stop <- w591 stop-if-true
        w584 = 5 ("Timeout (ms)")
        n289 = xnode "Invoke Method"("FPGA VI Reference In"=w590, "error in"=w589, "IRQ Number(s)"=i32[] [3, 25], "Timeout (ms)"=w584) -> ("FPGA VI Reference Out"=w573:refnum<k20>, "error out"=w572:errorcluster, "Timed Out"=w581:bool, "IRQ(s) Asserted"=w583:i32[])
        n290 = event shown="[0] Timeout" {
          selector: _ -> [_ _ _ _ _]
          dyn-events: _ -> [_ _ _ _ _]
          timeout: w584 -> [_ _ _ _ _]
          tunnel: w583 -> [w600 w607 w615 w623 w635]
          tunnel: [w599 w606 w614 w622 w634] -> w578
          tunnel: [w597 FALSE FALSE FALSE FALSE] -> w582
          tunnel: w573 -> [_ _ _ _ _]
          tunnel: w572 -> [_ _ _ _ _]
          tunnel: w571 -> [w595 _ _ _ _]
          event Timeout {
            n291 = event-data() -> ()  [unwired: 1 in, 2 out]
            n292 = local read "data_fetch_finished"() -> (w598:bool)
            n293 = Tick Count (ms)() -> (millisecond timer value=w596:u32)
            n294 = Subtract(x=w596, y=w595) -> (x-y=w594:u32)
            "x-y" <- w594
            n295 = Greater Or Equal?(x=w594, y=u32 60) -> (x >= y?=w592:bool)
            n296 = Implies(1:w598, 2:w592) -> (0:w597:bool)
            n297 = case shown="False" w597 {
              tunnel: w600 -> [w603 w604]
              tunnel: [w601 w604] -> w599
              frame False {
                n298 = Insert Into Array(array=w603, new element=26 ("new element/subarray")) -> (w601:i32[])  [unwired: 1 in]
              }
              frame True {
              }
            }
          }
          event "Move x": Value Change {
            n299 = event-data() -> ()  [unwired: 1 in, 2 out]
            n300 = case shown="True" "Move x" {
              tunnel: w607 -> [w609 w612]
              tunnel: [w609 w610] -> w606
              frame False {
              }
              frame True {
                n301 = Insert Into Array(array=w612, new element=9 ("new element/subarray")) -> (w610:i32[])  [unwired: 1 in]
              }
            }
          }
          event "Move y": Value Change {
            n302 = event-data() -> ()  [unwired: 1 in, 1 out]
            n303 = case shown="True" "Move y" {
              tunnel: w615 -> [w617 w620]
              tunnel: [w617 w618] -> w614
              frame False {
              }
              frame True {
                n304 = Insert Into Array(array=w620, new element=5 ("new element/subarray")) -> (w618:i32[])  [unwired: 1 in]
              }
            }
          }
          event "B-scan #", "Y Step Size": Value Change {
            n305 = event-data() -> ()  [unwired: 1 in, 1 out]
            n306 = local read "Manual y speed factor"() -> (w621:dbl)
            n307 = local read "Y Step Size"() -> (w629:dbl)
            n308 = local read "B-scan #"() -> (w630:dbl)
            n309 = Multiply(x=w630, y=w629) -> (x*y=w631:dbl)
            n310 = call "load_S_curve.vi"("pulses"=w631) -> ("Raw S Curve"=w628:dbl[])  [unwired: 9 in, 1 out]
            n311 = Multiply(x=w628, y=w621) -> (x*y=w627:dbl[])
            n312 = Round To Nearest(number=w627) -> (nearest integer value=w626:dbl[])
            n313 = To Long Integer(number=w626) -> (32bit integer=w625:i32[])
            n314 = local write "Bscan_Steps"(w625) -> ()
            n315 = Insert Into Array(array=w623, new element=7 ("new element/subarray")) -> (w622:i32[])  [unwired: 1 in]
          }
          event "Calc_delay": Value Change {
            n316 = event-data() -> ()  [unwired: 1 in, 1 out]
            n317 = case shown="True" "Calc_delay" {
              tunnel: w635 -> [w637 w639]
              tunnel: [w637 w638] -> w634
              frame False {
              }
              frame True {
                n318 = Insert Into Array(array=w639, new element=8 ("new element/subarray")) -> (w638:i32[])  [unwired: 1 in]
              }
            }
          }
        }
        n319 = And(x=w582, y=w581) -> (x .and. y?=w580:bool)
        n320 = Add Array Elements(numeric array=w578) -> (sum=w577:i32)
        n321 = case shown="False" w580 {
          tunnel: w578 -> [w660 _]
          tunnel: w573 -> [w650 w863]
          tunnel: [w659 w862] -> w588
          tunnel: w572 -> [w648 w861]
          tunnel: [w658 w860] -> w587
          tunnel: [w651 w839] -> w586
          tunnel: w577 -> [w657 _]
          tunnel: w576 -> [w656 w858]
          tunnel: [w654 w858] -> w585
          tunnel: w571 -> [w642 w850]
          tunnel: [w643 w851] -> w579
          frame False {
            n322 = local read "data_fetch_finished"() -> (w641:bool)
            n323 = Array Size(array=w660) -> (size(s)=w661:i32)
            n324 = Insert Into Array(array=w656, new element=w657) -> (w654:i32[])  [unwired: 1 in]
            n325 = local read "Bscan_Steps"() -> (w655:u32[])
            n326 = xnode "Read/Write Control"("FPGA VI Reference In"=w650, "error in"=w648) -> ("FPGA VI Reference Out"=w649:refnum<k20>, "error out"=w647:errorcluster, "stop"=w645:bool, "Tri_pt_sent"=w646:i32)
            n327 = And(x=w645, y=w641) -> (x .and. y?=w644:bool)
            n328 = case shown="False" w644 {
              tunnel: w661 -> [w670 _]
              tunnel: w660 -> [w669 _]
              tunnel: [w668 w828] -> w659
              tunnel: [w667 w827] -> w658
              tunnel: w655 -> [w666 _]
              tunnel: w649 -> [w665 w828]
              tunnel: w647 -> [w664 w827]
              tunnel: w646 -> [_ w826]
              tunnel: [w663 w824] -> w643
              tunnel: w642 -> [w662 w824]
              frame False {
                n329 = for {
                  N: w670 -> [_]
                  tunnel: w669 -> [w678] mode=indexing
                  tunnel: w666 -> [w676]
                  shift-right: [w677] -> w668
                  shift-left: w665 -> [w673]
                  shift-right: [w674] -> w667
                  shift-left: w664 -> [w675]
                  tunnel: [w672] -> w663
                  tunnel: w662 -> [w671]
                  n330 = case shown="25" w678 {
                    selector: w678 -> [_ w683 w692 _ _ _ _ w785 _]
                    tunnel: w673 -> [w681 w689 w698 w710 w731 w754 w764 w787 w807]
                    tunnel: [w681 w684 w694 w705 w730 w753 w758 w783 w807] -> w677
                    tunnel: w676 -> [_ w688 _ w706 w727 _ _ _ _]
                    tunnel: w675 -> [w680 w686 w695 w709 w728 w751 w763 w786 w806]
                    tunnel: [w680 w685 w693 w704 w729 w752 w757 w784 w806] -> w674
                    tunnel: [w679 w682 w690 w699 w722 w746 w755 w782 w805] -> w672
                    tunnel: w671 -> [w679 w682 w690 w699 w722 w746 w755 _ _]
                    frame 0, Default {
                    }
                    frame 2 {
                      n331 = xnode "Invoke Method"("FPGA VI Reference In"=w689, "Data"=w688) -> ("FPGA VI Reference Out"=w687:refnum<k20>)  [unwired: 2 in, 2 out]
                      n332 = xnode "Invoke Method"("FPGA VI Reference In"=w687, "error in"=w686, "IRQ Number(s)"=w683) -> ("FPGA VI Reference Out"=w684:refnum<k20>, "error out"=w685:errorcluster)
                    }
                    frame 4 {
                      n333 = local read "Vocie-coil Traj"() -> (w691:i16[])
                      n334 = xnode "Invoke Method"("FPGA VI Reference In"=w698, "error in"=w695, "Data"=w691) -> ("FPGA VI Reference Out"=w697:refnum<k20>, "error out"=w696:errorcluster)  [unwired: 1 in, 1 out]
                      n335 = xnode "Invoke Method"("FPGA VI Reference In"=w697, "error in"=w696, "IRQ Number(s)"=w692) -> ("FPGA VI Reference Out"=w694:refnum<k20>, "error out"=w693:errorcluster)
                    }
                    frame 9 {
                      # "Move x-axis by \"B-scan # x B-scan step size\""
                      n336 = flat-sequence {
                        tunnel: w710 -> [w716]
                        tunnel: w709 -> [w714]
                        tunnel: [w713] -> w703
                        tunnel: [w712] -> w702
                        tunnel: w703 -> [w719]
                        tunnel: w702 -> [w718]
                        tunnel: [w719] -> w701
                        tunnel: [w718] -> w700
                        tunnel: [w720] -> w707
                        tunnel: [w721] -> w708
                        tunnel: w701 -> [w721]
                        tunnel: w700 -> [w720]
                        frame #0 {
                          n337 = xnode "Read/Write Control"("FPGA VI Reference In"=w716, "error in"=w714, "Ele_Ini_Dir"="Left", "MnlMtrCtrl"=enum16{"Elevation Motor (y)", "Bscan Motor (x)"}."Bscan Motor (x)") -> ("FPGA VI Reference Out"=w713:refnum<k20>, "error out"=w712:errorcluster)
                        }
                        frame #1 {
                          n338 = Wait Until Next ms Multiple(millisecond multiple=u32 10) -> ()  [unwired: 1 out]
                        }
                        frame #2 {
                        }
                      }
                      n339 = xnode "Invoke Method"("FPGA VI Reference In"=w708, "error in"=w707, "Data"=w706) -> ("FPGA VI Reference Out"=w705:refnum<k20>, "error out"=w704:errorcluster)  [unwired: 1 in, 1 out]
                    }
                    frame 5 {
                      # "Move y-axis by \"B-scan # x B-scan step size\""
                      n340 = flat-sequence {
                        tunnel: w731 -> [w737]
                        tunnel: w728 -> [w736]
                        tunnel: [w740] -> w726
                        tunnel: [w739] -> w725
                        tunnel: w726 -> [w743]
                        tunnel: w725 -> [w742]
                        tunnel: [w743] -> w724
                        tunnel: [w742] -> w723
                        tunnel: [w744] -> w732
                        tunnel: [w745] -> w733
                        tunnel: w724 -> [w745]
                        tunnel: w723 -> [w744]
                        frame #0 {
                          n341 = local read "Ele_Ini_Dir"() -> (w735:bool)
                          n342 = Not(x=w735) -> (.not. x?=w734:bool)
                          n343 = xnode "Read/Write Control"("FPGA VI Reference In"=w737, "error in"=w736, "Ele_Ini_Dir"=w734, "MnlMtrCtrl"=enum16{"Elevation Motor (y)", "Bscan Motor (x)"}."Elevation Motor (y)") -> ("FPGA VI Reference Out"=w740:refnum<k20>, "error out"=w739:errorcluster)
                        }
                        frame #1 {
                          n344 = Wait Until Next ms Multiple(millisecond multiple=u32 10) -> ()  [unwired: 1 out]
                        }
                        frame #2 {
                        }
                      }
                      n345 = xnode "Invoke Method"("FPGA VI Reference In"=w733, "error in"=w732, "Data"=w727) -> ("FPGA VI Reference Out"=w730:refnum<k20>, "error out"=w729:errorcluster)  [unwired: 1 in, 1 out]
                    }
                    frame 7 {
                      n346 = local read "Y Step Size"() -> (w749:dbl)
                      n347 = local read "B-scan #"() -> (w750:dbl)
                      n348 = Multiply(x=w750, y=w749) -> (x*y=w748:dbl)
                      n349 = Add(x=w748, y=w748) -> (x+y=w747:dbl)
                      n350 = xnode "Invoke Method"("FPGA VI Reference In"=w754, "error in"=w751, "Depth"=w747) -> ("FPGA VI Reference Out"=w753:refnum<k20>, "error out"=w752:errorcluster)
                    }
                    frame 8 {
                      n351 = local read "VC_POS"() -> (w767:i16[])
                      n352 = Array Max & Min(array=w767) -> (max value=w780:i16, min value=w779:i16)  [unwired: 2 out]
                      n353 = call-poly <vilib>:"Normalize.vi"("Vector"=w767) -> ("Normalized Vector"=w766:dbl[])  [unwired: 1 in, 3 out]
                      n354 = local read "VC_In"() -> (w778:dbl[])
                      n355 = Subtract(x=w780, y=w779) -> (x-y=→"VC range":i16)
                      n356 = call "Calc Phase Shift.vi"("Signal 2"=w766, "Signal 1"=w778) -> ("Phase Shift"=w776:dbl)  [unwired: 6 in, 3 out]
                      "Phase Shift" <- w776
                      n357 = local read "Phase0(deg)"() -> (w777:dbl)
                      n358 = local read "VCsamples"() -> (w759:i32)
                      n359 = local read "signal type"() -> (w769:T1)
                      n360 = Subtract(x=w777, y=w776) -> (x-y=w768:dbl)
                      n361 = local read "x0 (mm)"() -> (w772:dbl)
                      n362 = local write "Phase0(deg)"(w768) -> ()
                      n363 = local read "x (mm)"() -> (w771:dbl)
                      n364 = call <vilib>:"Signal Generator by Duration.vi"("signal type"=w769, "reset phase"=TRUE, "# of samples"=w759, "frequency"=1.0, "amplitude"=w771, "dc offset"=w772, "phase in"=w768) -> ("signal"=w774:dbl[])  [unwired: 5 in, 3 out]
                      n365 = Multiply(x=w774, y=3276.8 ("frequency")) -> (x*y=w775:dbl[])
                      n366 = To Word Integer(number=w775) -> (16bit integer=w762:i16[])
                      n367 = local write "Vocie-coil Traj"(w762) -> ()
                      n368 = xnode "Invoke Method"("FPGA VI Reference In"=w764, "error in"=w763, "Data"=w762) -> ("FPGA VI Reference Out"=w760:refnum<k20>, "error out"=w761:errorcluster)  [unwired: 1 in, 1 out]
                      n369 = xnode "Read/Write Control"("FPGA VI Reference In"=w760, "error in"=w761, "VC_pt_in_fifo"=w759) -> ("FPGA VI Reference Out"=w758:refnum<k20>, "error out"=w757:errorcluster)
                    }
                    frame 25 {
                      n370 = xnode "Invoke Method"("FPGA VI Reference In"=w787, "error in"=w786, "IRQ Number(s)"=w785) -> ("FPGA VI Reference Out"=w783:refnum<k20>, "error out"=w784:errorcluster)
                      n371 = case shown="True" "acc_PA" {
                        frame False {
                        }
                        frame True {
                          n372 = local read "DataQueue"() -> (w790:refnum<queue>)
                          n373 = local read "ALAZAR9350"() -> (w794:i32)
                          n374 = call "ATS_AsyncDMA_Device.vi"("DeviceIn"=w794, "ATS_Async_Ctrl"=ATS_Async_Ctrl."Get", "WaitTimeOut (ms)"=u32 100) -> ("Buffer"=w789:u16[], "Async_Status"=w799:T9, "Return Code"=w796:u32)  [unwired: 5 in, 5 out]
                          n375 = Enqueue Element(queue=w790, element=w789) -> ()  [unwired: 2 in, 3 out]
                          n376 = Unbundle By Name(w799) -> ("Valid"=w792:bool, "Completed"=w801:bool, "Start DMA"=w803:bool, "Timeout"=w802:bool, "Error"=w800:bool)
                          n377 = call "ATS_ErrorCode.vi"("ErrorCode"=w796) -> ("error out"=w797:errorcluster)  [unwired: 1 in, 5 out]
                          n378 = Unbundle By Name(w797) -> ("source"=→"Error source":string)
                          n379 = Compound Arithmetic op=OR(invert w792, w801, invert w803, w802, w800) -> (→"DAQ Error":bool)
                        }
                      }
                      n380 = local write "save_rate"(u32 40 ("save_rate")) -> ()
                      n381 = Tick Count (ms)() -> (millisecond timer value=w782:u32)
                    }
                    frame 26 {
                      n382 = local read "acc_PA"() -> (w808:bool)
                      n383 = case shown="True" w808 {
                        frame False {
                        }
                        frame True {
                          # "Fetch data on software interupt"
                          n384 = local read "ALAZAR9350"() -> (w812:i32)
                          n385 = local read "DataQueue"() -> (w811:refnum<queue>)
                          n386 = call "ATS_AsyncDMA_Device.vi"("DeviceIn"=w812, "ATS_Async_Ctrl"=ATS_Async_Ctrl."Get", "WaitTimeOut (ms)"=u32 100) -> ("Buffer"=w810:u16[], "Async_Status"=w816:T9, "Return Code"=w813:u32)  [unwired: 5 in, 5 out]
                          n387 = Unbundle By Name(w816) -> ("Valid"=w817:bool, "Completed"=w819:bool, "Start DMA"=w821:bool, "Timeout"=w820:bool, "Error"=w818:bool)
                          n388 = call "ATS_ErrorCode.vi"("ErrorCode"=w813) -> ("error out"=w814:errorcluster)  [unwired: 1 in, 5 out]
                          n389 = Enqueue Element(queue=w811, element=w810) -> ()  [unwired: 2 in, 3 out]
                          n390 = Unbundle By Name(w814) -> ("source"=w815:string)
                          n391 = Compound Arithmetic op=OR(invert w817, w819, invert w821, w820, w818) -> (w809:bool)
                          n392 = local write "Error source"(w815) -> ()
                          n393 = local write "DAQ Error"(w809) -> ()
                        }
                      }
                      n394 = local write "save_rate"(u32 10 ("save_rate")) -> ()
                      n395 = Tick Count (ms)() -> (millisecond timer value=w805:u32)
                    }
                  }
                }
              }
              frame True {
                n396 = local read "Aline Stop #"() -> (w825:i32)
                n397 = Equal?(x=w826, y=w825) -> ()  [unwired: 1 out]
              }
            }
            n398 = local read "DAQ Error"() -> (w652:bool)
            n399 = Or(x=FALSE ("stop"), y=w652) -> (x .or. y?=w651:bool)
          }
          frame True {
            n400 = xnode "Read/Write Control"("FPGA VI Reference In"=w863, "error in"=w861) -> ("FPGA VI Reference Out"=w862:refnum<k20>, "error out"=w860:errorcluster, "stop"=w847:bool, "Tri_pt_sent"=w848:i32, "Ele_pt_sent"=→"Ele_pt_sent":i32, "B-Scan Pos"=→"B-Scan Pos":i32, "x step motor pos"=→"x step motor pos":i32)  [unwired: 1 out]
            "Tri_pt_sent" <- w848
            "vc_pt_sent" <- w848
            n401 = local read "Aline Stop #"() -> (w845:i32)
            n402 = Tick Count (ms)() -> (millisecond timer value=w852:u32)
            n403 = Subtract(x=w852, y=w850) -> (x-y=w855:u32)
            n404 = local read "Y Enable"() -> (w835:bool)
            n405 = Equal?(x=w848, y=w845) -> (x = y?=w849:bool)
            n406 = Greater Or Equal?(x=w855, y=u32 200) -> (x >= y?=w853:bool)
            n407 = local read "catbscan"() -> (w831:i16)
            n408 = And(x=w835, y=w849) -> (x .and. y?=w846:bool)
            n409 = local read "B-scan #"() -> (w836:dbl)
            n410 = local read "B-scan saved"() -> (w832:i32)
            n411 = case shown="True" w853 {
              tunnel: w852 -> [_ _]
              tunnel: [w864 w865] -> w851
              tunnel: w850 -> [w864 w865]
              frame False {
              }
              frame True {
              }
            }
            n412 = local read "3D scan #"() -> (w838:dbl)
            n413 = Or(x=w847, y=w846) -> (x .or. y?=w840:bool)
            n414 = Multiply(x=w831, y=1) -> (x*y=w830:i32)
            n415 = local read "Save Data"() -> (w844:bool)
            n416 = Multiply(x=w838, y=w836) -> (x*y=w837:dbl)
            n417 = Add(x=w832, y=w830) -> (x+y=w833:i32)
            n418 = Subtract(x=w837, y=w833) -> (x-y=w843:dbl)
            n419 = Boolean To (0,1)(Boolean=w844) -> (0, 1=w842:i16)
            n420 = Multiply(x=w843, y=w842) -> (x*y=w834:dbl)
            n421 = Less Or Equal To 0?(x=w834) -> (x <= 0?=w841:bool)
            "data_fetch_finished" <- w841
            n422 = And(x=w840, y=w841) -> (x .and. y?=w839:bool)
          }
        }
        n423 = Or(x="stop", y=w586) -> (x .or. y?=w591:bool)
        "stop_disp" <- w591
      }
      n424 = while {
        stop <- w445 stop-if-true
        n425 = local read "DataQueue"() -> (w451:refnum<queue>)
        n426 = local read "stop_disp"() -> (w447:bool)
        n427 = Get Queue Status(queue=w451) -> (queue out=w449:refnum<queue>, # elements in queue=w448:i32)  [unwired: 2 in, 6 out]
        n428 = Wait Until Next ms Multiple(millisecond multiple="save_rate") -> ()  [unwired: 1 out]
        n429 = Equal To 0?(x=w448) -> (x = 0?=w446:bool)
        n430 = And(x=w446, y=w447) -> (x .and. y?=w445:bool)
        n431 = Greater Than 0?(x=w448) -> (x > 0?=w450:bool)
        n432 = case shown="True" w450 {
          tunnel: w449 -> [_ w458]
          frame False {
            n433 = Wait Until Next ms Multiple(millisecond multiple=u32 5) -> ()  [unwired: 1 out]
          }
          frame True {
            n434 = local read "B-scan saved"() -> (w463:i32)
            n435 = Dequeue Element(queue=w458) -> (element=w455:u16[])  [unwired: 2 in, 3 out]
            n436 = And(x=w463, y="EveryFrm") -> (x .and. y?=w459:i32)
            n437 = Equal To 0?(x=w459) -> (x = 0?=w460:bool)
            n438 = And(x="Display Data Per             Frm", y=w460) -> (x .and. y?=w461:bool)
            n439 = case shown="True" w461 {
              tunnel: w455 -> [_ w469]
              tunnel: [u16[] [] w468] -> w453
              frame False {
              }
              frame True {
                n440 = local read "B-scan displayed"() -> (w478:i32)
                n441 = local read "catbscan"() -> (w475:i16)
                n442 = local read "catbscan"() -> (w470:i16)
                n443 = local read "Alines"() -> (w473:i32)
                n444 = local read "Ch1 Pt"() -> (w476:i32)
                n445 = Multiply(x=w476, y=w475) -> (x*y=w474:i32)
                n446 = Multiply(x=w470, y=w473) -> (x*y=w471:i32)
                n447 = local read "Pt per A-line"() -> (w472:i32)
                n448 = Split 1D Array(array=w469, index=w474) -> (first subarray=w480:u16[])  [unwired: 1 out]
                n449 = Reshape Array(w480, w471, w472) -> (w466:u16[][])
                n450 = case shown="True" "A/B-line show" {
                  tunnel: w469 -> [_ w482]
                  tunnel: w466 -> [_ w481]
                  frame False {
                  }
                  frame True {
                    "PD" <- w482
                    "B-Scan" <- w481
                  }
                }
                n451 = Add(x=w470, y=w478) -> (x+y=w477:i32)
                n452 = local write "B-scan displayed"(w477) -> ()
                n453 = case shown="True" "MAP Disp" {
                  tunnel: w471 -> [_ w502]
                  tunnel: w478 -> [_ w501]
                  tunnel: w466 -> [_ w500]
                  tunnel: [u16[] [] w487] -> w468
                  frame False {
                  }
                  frame True {
                    n454 = local read "B-scan #"() -> (w493:dbl)
                    n455 = for {
                      N: w502 -> [_]
                      tunnel: w500 -> [w521] mode=indexing
                      tunnel: [w516] -> w487 mode=indexing
                      n456 = Array Subset(array=w521, index="start", length="depth") -> (w520:u16[])
                      n457 = Array Max & Min(array=w520) -> (max value=w517:u16, min value=w515:u16)  [unwired: 2 out]
                      n458 = Subtract(x=w517, y=w515) -> (x-y=w516:u16)
                    }
                    n459 = local read "catbscan"() -> (w492:i16)
                    n460 = local read "Alines"() -> (w491:i32)
                    n461 = Subtract(x=w493, y=1) -> (x-y=w497:dbl)
                    n462 = Reshape Array(w487, w492, w491) -> (w488:u16[][])
                    n463 = Quotient & Remainder(x=w501, y=w493) -> (x-y*floor(x/y)=w496:dbl, floor(x/y)=w499:dbl)
                    n464 = Subtract(x=w497, y=w496) -> (x-y=w495:dbl)
                    n465 = And(x=w499, y=1) -> (x .and. y?=w494:i32)
                    n466 = Transpose 2D Array(2D array=w488) -> (transposed array=w490:u16[][])
                    n467 = Greater Than 0?(x=w494) -> (x > 0?=w486:bool)
                    n468 = And(x=w486, y="showmap") -> (x .and. y?=w484:bool)
                    n469 = case shown="True" w484 {
                      tunnel: w490 -> [w503 w512]
                      tunnel: w496 -> [_ w510]
                      tunnel: w495 -> [w504 _]
                      frame False {
                        n470 = disable-structure shown="Disabled" {
                          disable-tunnel: w504 -> [w506 _]
                          disable-tunnel: w503 -> [w505 _]
                          frame Disabled {
                            n471 = local read "MAP"() -> (w508:dbl[][])
                            n472 = Replace Array Subset(array=w508, new element=w505, index (row)=0 ("disabled index (row)"), index (col)=w506) -> (w509:dbl[][])
                            n473 = local write "MAP"(w509) -> ()
                          }
                          frame Enabled {
                          }
                        }
                      }
                      frame True {
                        n474 = local read "MAP"() -> (w513:dbl[][])
                        n475 = Replace Array Subset(array=w513, new element=w512, index (row)=0 ("disabled index (row)"), index (col)=w510) -> (w514:dbl[][])
                        n476 = local write "MAP"(w514) -> ()
                      }
                    }
                  }
                }
              }
            }
            n477 = Select(t=w453, s="Savemap", f=w455) -> (s? t:f=w454:u16[])
            n478 = case shown="True" "Save Data" {
              tunnel: w454 -> [_ w522]
              frame False {
              }
              frame True {
                n479 = local read "B-scan saved"() -> (w524:i32)
                n480 = local read "catbscan"() -> (w523:i16)
                n481 = local read "file_ref"() -> (w527:refnum<file>)
                n482 = Add(x=w524, y=w523) -> (x+y=w525:i32)
                n483 = local write "B-scan saved"(w525) -> ()
                n484 = Write to Binary File(file (use dialog)=w527, data=w522, 5:FALSE ("prepend array or string size? (T)"), 9:T4."native, host order" ("byte order (0:big-endian, network order)")) -> (error out=w526:errorcluster)  [unwired: 1 in, 3 out]
                n485 = call <vilib>:"Simple Error Handler.vi"("error in (no error)"=w526) -> ()  [unwired: 4 in, 5 out]
              }
            }
          }
        }
      }
      n486 = xnode "Read/Write Control"("FPGA VI Reference In"=w434, "error in"=w433, "stop"=TRUE, "Ele_StepM_En"=FALSE, "Bscan_StepM_En"=FALSE) -> ("FPGA VI Reference Out"=w431:refnum<k20>, "error out"=w430:errorcluster, "Ele_pt_sent"=w414:i32, "B-Scan Pos"=w409:i32, "Tri_pt_sent"=w377:i32)
      n487 = local write "B-Scan Pos"(w409) -> ()
      n488 = local write "Ele_pt_sent"(w414) -> ()
      n489 = local write "Tri_pt_sent"(w377) -> ()
      n490 = local write "vc_pt_sent"(w377) -> ()
      n491 = xnode "Close FPGA VI Reference"("FPGA VI Reference In"=w431, "error in"=w430) -> ("error out"=w429:errorcluster)
      n492 = call <vilib>:"Simple Error Handler.vi"("error in (no error)"=w429) -> ()  [unwired: 4 in, 5 out]
    }
    frame #3 {
      n493 = local read "DataQueue"() -> (w869:refnum<queue>)
      n494 = local read "ALAZAR9350"() -> (w868:i32)
      n495 = local read "file_ref"() -> (w867:refnum<file>)
      n496 = Release Queue(queue=w869) -> ()  [unwired: 2 in, 3 out]
      n497 = Close File(refnum=w867) -> ()  [unwired: 1 in, 2 out]
      n498 = call "ATS_Device.vi"("DevCtrl"=Device_Ctrl."Abort", "DeviceIn"=w868) -> ()  [unwired: 3 in, 7 out]
    }
    frame #4 {
    }
  }
